vi "Dashboard Main.vi"() -> ()   [LabVIEW 2016]
uses:
  <vilib>/Utility/miscctls.llb/LVRowAndColumnTypeDef.ctl
  <vilib>/event_ctls.llb/eventvkey.ctl
  <vilib>/Rock Robotics/Network Tables/NT Read Numeric Array.vi
  <vilib>/Rock Robotics/Network Tables/NT Read Boolean.vi
  <vilib>/Rock Robotics/Network Tables/NT Write Boolean.vi
  <vilib>/Rock Robotics/Network Tables/NT Read Boolean Array.vi
  <vilib>/Utility/file.llb/Read Delimited Spreadsheet (string).vi
  <vilib>/Utility/file.llb/Read Delimited Spreadsheet (DBL).vi
  <vilib>/Rock Robotics/Network Tables/NT Write String Array.vi
  <vilib>/Utility/file.llb/Write Delimited Spreadsheet (string).vi
  <vilib>/Rock Robotics/Network Tables/NT Write Numeric Array.vi
  <vilib>/Utility/file.llb/Write Delimited Spreadsheet (DBL).vi
  <vilib>/Rock Robotics/WPI/Dashboard/WPI_DashboardLogging Global.vi
panel:
  in  "Camera Settings Right":T1={"Frame Rate"=15, "Compression"=30, "Size"=1, "DB Camera Config"=FALSE} {"Frame Rate" scale=1.0..30.0; "Compression" scale=100.0..-1.0; "Size" items=["640x480", "320x240", "160x120"]}
  in  "Camera Name Right":string(combo)="No Camera Selection"
  out "Camera Info":cluster{"Mbps LED":bool, "Mbps":dbl, "fps":dbl} {"fps" format="%#.1g"; "Mbps" format="%#.1g"}
  in  "Camera Settings":T1={"Frame Rate"=15, "Compression"=30, "Size"=1, "DB Camera Config"=FALSE} {"Frame Rate" scale=1.0..30.0; "Compression" scale=100.0..-1.0; "Size" items=["640x480", "320x240", "160x120"]}
  in  "TCP":refnum<k5>
  in  "Rec Mode":enum32{"Stop", "Record", "Playback"}(radio)
  out "Robot IP":string="0.0.0.0"
  out "Image Message":string="Timeout in Camera Communications"
  in  "Dashboard Tab":T2(tab)=enum."Config"
  in  "Disable Drop Ropes":bool
  out "Shoot RPM":dbl format="%#_10f"
  in  "Config File Path":path=path "C:/Users/Admin/Desktop/ConfigCSV.csv"
  in  "Slow Drive":dbl=50.0
  in  "Fast Drive":dbl=100.0
  out "Shoot PWM":dbl
  in  "Thump Interval":dbl=0.4
  out "Pixy Height":dbl
  out "Pixy Width":dbl
  out "Pixy X":dbl
  in  "Lock Servo B":dbl=170.0
  in  "Lock Servo A":dbl
  out "Move":dbl=85.0
  out "Zero":dbl=77.0
  in  "Gear Servo Values":u16(ring) items=["A Values | Comp", "B Values | Practice"]
  in  "Gear Servo Move B":dbl=85.0
  in  "Gear Servo Move A":dbl=85.0
  in  "Gear Servo Zero B":dbl=79.5
  in  "Gear Servo Zero A":dbl=77.0
  out "Notify 2":string="NT Disconnected"
  out "Verify 2":string="No Comm"
  in  "Time Remain":bool=TRUE
  out "Auto Ran":string="Not Available"
  out "Code Version":string="Not Available"
  out "NT Connection":bool
  out "MotorChart R":cluster{"Numeric":dbl, "Numeric":dbl}(graph)
  out "MotorChart L":cluster{"Numeric":dbl, "Numeric":dbl}(graph)
  out "MotorSliders R":cluster{"MotorSlide1":dbl, "MotorSlide2":dbl} {"MotorSlide2" scale=-1.0..1.0 scale format="%#_2e"; "MotorSlide1" scale=-1.0..1.0 scale format="%#_2e"}
  out "MotorSliders L":cluster{"MotorSlide1":dbl, "MotorSlide2":dbl} {"MotorSlide2" scale=-1.0..1.0 scale format="%#_2e"; "MotorSlide1" scale=-1.0..1.0 scale format="%#_2e"}
  out "JS1 Z":dbl(slide) scale=-1.0..1.0 scale format="%#_2e"
  out "JS1 Graph":cluster{"X":dbl, "Y":dbl}[](graph)
  out "JS1 Buttons":T3
  out "JS2 Z":dbl(slide) scale=-1.0..1.0 scale format="%#_2e"
  out "JS2 Graph":cluster{"X":dbl, "Y":dbl}[](graph)
  out "JS2 Buttons":T3
  out "Mode":T4(ring)=enum."Disconnected"
  in  "Auto Array File Path":path=path "C:/Users/Admin/Desktop/AutoCSV.csv"
  out "Camera Image Right":T5(plugin-control)
  out "Climb Inverted":bool
  in  "Auto Gear Timeout":dbl=-1.0
  out "Shoot Toggle":bool
  in  "Auto Turn Speed":dbl=0.4
  out "Gear Box Stat":bool
  in  "Auto Drive Speed":dbl=0.5
  in  "RPM 4":dbl=0.85
  in  "RPM 3":dbl=0.95
  in  "RPM 2":dbl=0.9
  in  "Serializer Speed":dbl=0.8
  out "Gear Plate":bool
  in  "Pixy Center":dbl=-2.3
  in  "RPM 1":dbl=1.0 min=0.0 max=1.0
  in  "Climb Speed":dbl=1.0
  in  "Slow Turn":dbl=50.0
  in  "Fast Turn":dbl=100.0
  in  "Auto Select":string(combo)="Default"
  out "Pixy Object Stat":bool
  out "Time Remaining":dbl=135.0 format="%#.0f"
  out "PDP Comm":string="Code Ver : Not Available"
  out "PDP Comm":bool=TRUE
  out "Notifyer":bool
  out "Notifyer Box":string="ERROR - DS is not Running"
  out "Auto Ready":bool
  out "Verify":string="Auto Ran : Not Available"
  in  "Position":string(combo)="Default"
  out "Gear Status":bool
  out "Channel 8":bool
  out "Channel 7":bool
  out "Channel 6":bool
  out "Channel 5":bool
  out "Channel 10":bool
  out "Channel 9":bool
  out "Channel 4":bool
  out "Channel 11":bool
  out "Channel 3":bool
  out "Channel 1":bool
  out "Channel 0":bool
  out "Channel 2":bool
  out "Channel 11":dbl
  out "Channel 10":dbl
  out "Channel 9":dbl
  out "Channel 8":dbl
  out "Channel 7":dbl
  out "Channel 6":dbl
  out "Channel 5":dbl
  out "Channel 4":dbl
  out "Channel 3":dbl
  out "Channel 2":dbl
  out "Channel 1":dbl
  out "Channel 15":bool
  out "Channel 14":bool
  out "Channel 13":bool
  out "Channel 12":bool
  out "Channel 15":dbl
  out "Channel 14":dbl
  out "Channel 13":dbl
  out "Channel 12":dbl
  out "Channel 0":dbl
  in  "Reset Sticky":bool
  in  "Reset Latched":bool
  out "Config Saved":bool
  in  "Update Config":bool
  in  "ARM Write":bool
  in  "Read Config":bool
  in  "Config Cluster":T6={"a"=0.0, "b"=0.0, "c"=0.0, "d"=0.0, "h"=0.0, "proportional gain (Kc)"=0.019, "integral time (Ti, min)"=0.0, "derivative time (Td, min)"=0.0, "Fast Speed"=-0.3, "setpoint"=1400.0, "Approach Speed"=-0.12, "proportional gain (Kc) 2"=0.052, "integral time (Ti, min) 2"=0.0, "derivative time (Td, min) 2"=0.002, "Cutoff Delay"=0.5, "Sense Delay"=0.0, "Wait Till Shoot"=0.0, "proportional gain (Kc) 3"=0.0, "integral time (Ti, min) 3"=0.0, "derivative time (Td, min) 3"=0.0, "Aim Offset"=0.0, "PWM Offset"=0.0} {"derivative time (Td, min) 3" format="%.3f"; "integral time (Ti, min) 3" format="%.3f"; "proportional gain (Kc) 3" format="%.3f"; "Cutoff Delay" min=0.0; "derivative time (Td, min)" format="%.3f"; "integral time (Ti, min)" format="%.3f"; "proportional gain (Kc)" format="%.3f"; "derivative time (Td, min) 2" format="%.3f"; "integral time (Ti, min) 2" format="%.3f"; "proportional gain (Kc) 2" format="%.3f"}
  in  "Test Slider":dbl(slide) scale=0.0..100.0 scale format="%#_3g"
  in  "On/Off":bool caption="Solenoid"
  in  "Test Name":u16(ring) items=["Select the test to run..."]
  in  "Test Tree":string(tree)
  in  "Motor":cluster{"Value":dbl, "Enable":bool} {"Value" scale=-1.0..1.0 scale format="%#_3g"}
  out "Progress":T7 {"Test Progress" scale=0.0..100.0}
  in  "Rev/Fwd":cluster{"Forward":bool, "Reverse":bool}
  in  "Test Ring":u16(ring) items=["Monochrome", "Color"]
  out "Cmd Status":string
  in  "Execute Command":bool
  in  "Command Params":string[][](table)
  in  "Command Selection":i32(listbox)
  out "Saved to Sheet":bool
  in  "ARM Overwrite":bool
  in  "Read Sheet":bool
  in  "Update Sheet":bool
  in  "Auto Array":string[][](array[string])
  in  "CheckList":i32(listbox)
  out "Tree":string(tree)
  out "Camera Image":T5(plugin-control)
  out "Background":bool
  in  "Camera Name":string(combo)="No Camera Selection"
  # "HW"
  # "HW"
  # "Joysticks"
  # "Drive Motors"
  # "Front"
  # "Right"
  # "Left"
  # "Back"
  # "Manual PWM"
  # "Drivetrain"
  # "Shooter"
  # "Climbing"
  # "Serializer"
  # "Unused"
  # "Feeder"
  # "Intake"
  # "Shooting Coefficents"
  # "Gear Aiming PID Gains"
  # "Other Gear Aiming Stuff"
  # "Shooting Aiming PID Gains"
  # "Other Shooting Stuff"
  # "More Shooting Stuff"
  # "Shoot Wheel PID Gains"
  # "Format: [Command] [Time in Tenths]"
  # "Label         Move 1       Rot 1         Act 1        Move 2       Rot 2        Move 3       Act 2"
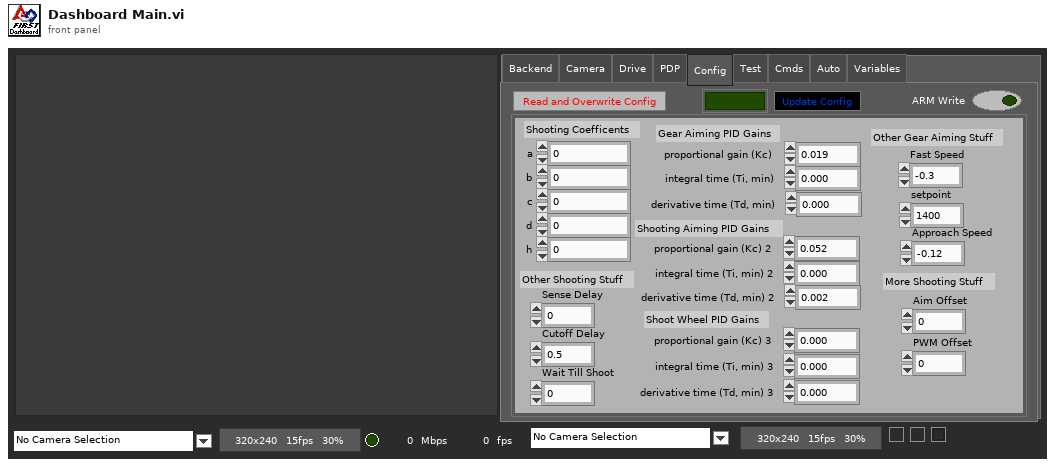
[diagram p1: front panel]
types:
  T1 = cluster{"Frame Rate":i32, "Compression":i32, "Size":u16, "DB Camera Config":bool}
  T2 = enum32{"Backend", "Camera", "Drive", "PDP", "Config", "Test", "Cmds", "Auto", "Variables"}
  T3 = cluster{bool, bool, bool, bool, bool, bool, bool, bool, bool, bool, bool, bool}
  T4 = enum8{"Tele-Op Disabled", "Tele-Op Enabled", "Auto Disabled", "Auto Enabled", "Test Disabled", "Test Enabled", "Disconnected", "No Code", "E-Stop"}
  T5 = typedef "IMAQ Image.ctl" = refnum<image>
  T6 = cluster{"a":dbl, "b":dbl, "c":dbl, "d":dbl, "h":dbl, "proportional gain (Kc)":dbl, "integral time (Ti, min)":dbl, "derivative time (Td, min)":dbl, "Fast Speed":dbl, "setpoint":dbl, "Approach Speed":dbl, "proportional gain (Kc) 2":dbl, "integral time (Ti, min) 2":dbl, "derivative time (Td, min) 2":dbl, "Cutoff Delay":dbl, "Sense Delay":dbl, "Wait Till Shoot":dbl, "proportional gain (Kc) 3":dbl, "integral time (Ti, min) 3":dbl, "derivative time (Td, min) 3":dbl, "Aim Offset":dbl, "PWM Offset":dbl}
  T7 = cluster{"Test Progress":u8, "Test Progress Text":string}
  T8 = typedef "Image Type" = u32
  T9 = cluster{"IDs":cluster{"RPC field ID":u16, "Unique ID":u16}, "String":string}
  T10 = enum32{"Drive", "Basic", "Custom", "Test", "Checklist", "Variables"}
  T11 = cluster{"all rows[0]":dbl, "all rows[1]":dbl, "all rows[2]":dbl, "all rows[3]":dbl, "all rows[4]":dbl, "all rows[5]":dbl, "all rows[6]":dbl, "all rows[7]":dbl, "all rows[8]":dbl, "all rows[9]":dbl, "all rows[10]":dbl, "all rows[11]":dbl, "all rows[12]":dbl, "all rows[13]":dbl, "all rows[14]":dbl, "all rows[15]":dbl, "all rows[16]":dbl, "all rows[17]":dbl, "all rows[18]":dbl, "all rows[19]":dbl, "all rows[20]":dbl, "all rows[21]":dbl}
  T12 = cluster{"Error Strings":string, "Disable Counts":cluster{u16, u16}, "Rail Faults":cluster{u16, u16, u16}, "Robot IP":string, "DB Mode":u8, "Event Info":cluster{"Name":string, "Type":u8, "Number":u16, "Replay":u8}}
  T13 = cluster{"Storage":cluster{"Disk Free":u64, "RAM Block":u32, "RAM free":u32}, "CPU Utilization":cluster{"CPU % ISR":sgl, "CPU % Time Crit":sgl, "CPU % Timed Str":sgl, "CPU % High":sgl, "CPU % Above":sgl, "CPU % Normal":sgl, "CPU % Low":sgl}, "CAN":cluster{"% Bus Utilization":sgl, "Bus Off Cnt":u32, "TX_FIFO Full Cnt":u32, "Receive Error Cnt":u8, "Transmit Error Cnt":u8}, "HID":cluster{"HID Outputs":u32, "Rumble Low":u16, "Rumble High":u16}[]}
  T14 = cluster{"Status bits":cluster{"Test Mode":bool, "Autonomous":bool, "Enabled":bool, "Code Start":bool, "Brownout":bool, "Reserved 2":bool, "Reserved 3":bool, "E-Stop":bool}, "Code Trace":cluster{"Disabled":bool, "TeleOp":bool, "Auto":bool, "Test":bool}, "Controller Type":enum16{"unknown", "cRIO", "roboRio"}, "Code?":enum16{"unknown", "noCode", "code"}, "Battery V":dbl}
  T15 = cluster{"Control Bits":cluster{"TestMode":bool, "Autonomous":bool, "Enabled":bool, "FMS Present":bool, bool, bool, bool, "E-Stop":bool}, "Team Station ":u8, "Countdown":sgl, "Joystick Values":cluster{"Axes":dbl[], "Buttons":bool[], "POVs":i16[]}[]}
  T16 = cluster{"Axes":dbl[], "Buttons":bool[], "POVs":i16[]}[]
  T17 = cluster{"Axes":dbl[], "Buttons":bool[], "POVs":i16[]}
  T18 = cluster{"Buttons[0]":bool, "Buttons[1]":bool, "Buttons[2]":bool, "Buttons[3]":bool, "Buttons[4]":bool, "Buttons[5]":bool, "Buttons[6]":bool, "Buttons[7]":bool, "Buttons[8]":bool, "Buttons[9]":bool, "Buttons[10]":bool, "Buttons[11]":bool}
  T19 = cluster{"Camera Image":refnum<vi>, "Dashboard Tab":refnum<vi>, "Background":refnum<vi>, "Rec Mode":refnum<vi>, "Test Slider":refnum<vi>, "On/Off ":refnum<vi>, "Test Ring":refnum<vi>, "Rev/Fwd":refnum<vi>, "Test Name":refnum<vi>, "Motor":refnum<vi>, "Progress":refnum<vi>, "CheckList":refnum<vi>, "Tree":refnum<vi>, "Test Tree":refnum<vi>, "Command Params":refnum<vi>, "Command Selection":refnum<vi>, "Execute Command":refnum<vi>, "Cmd Status":refnum<vi>, "Camera Settings":refnum<vi>, "Camera Name":refnum<vi>, "Camera Info":refnum<vi>, "Camera Settings Right":refnum<vi>, "Camera Name Right":refnum<vi>, "Camera Image Right":refnum<vi>}
  T20 = cluster{"Operation":enum16{"Update", "Clear"}, "Color Box":u32}[]
  T21 = typedef "eventvkey.ctl" = enum16{"ASCII", "Enter", "Return", "Shift", "Ctrl", "Alt", "Cmd", "Opt", "Caps", "NumLock", "Clear", "Break", "Up", "Down", "Left", "Right", "Insert", "Delete", "Home", "End", "PageUp", "PageDown", "Escape", "Help", "Pause", "ScrollLock", "F1", "F2", "F3", "F4", "F5", "F6", "F7", "F8", "F9", "F10", "F11", "F12", "F13", "F14", "F15", "F16", "F17", "F18", "F19", "F20", "F21", "F22", "F23", "F24", "Play", "VolumeUp", "VolumeDown", "Mute", "Two Byte Char"}
  T22 = cluster{"Image Size":bool, "Image Type":bool, "Pixel Value":bool, "ROI Information":bool, "Zoom Factor":bool}
  T23 = cluster{"Operation":enum16{"Update", "Clear"}, "Color Box":u32}
  T24 = typedef "LVRowAndColumnTypeDef.ctl" = cluster{"Row":i32, "Column":i32}
  T25 = cluster{"Shift":bool, "Ctrl":bool, "Alt":bool, "Cmd":bool, "Opt":bool}
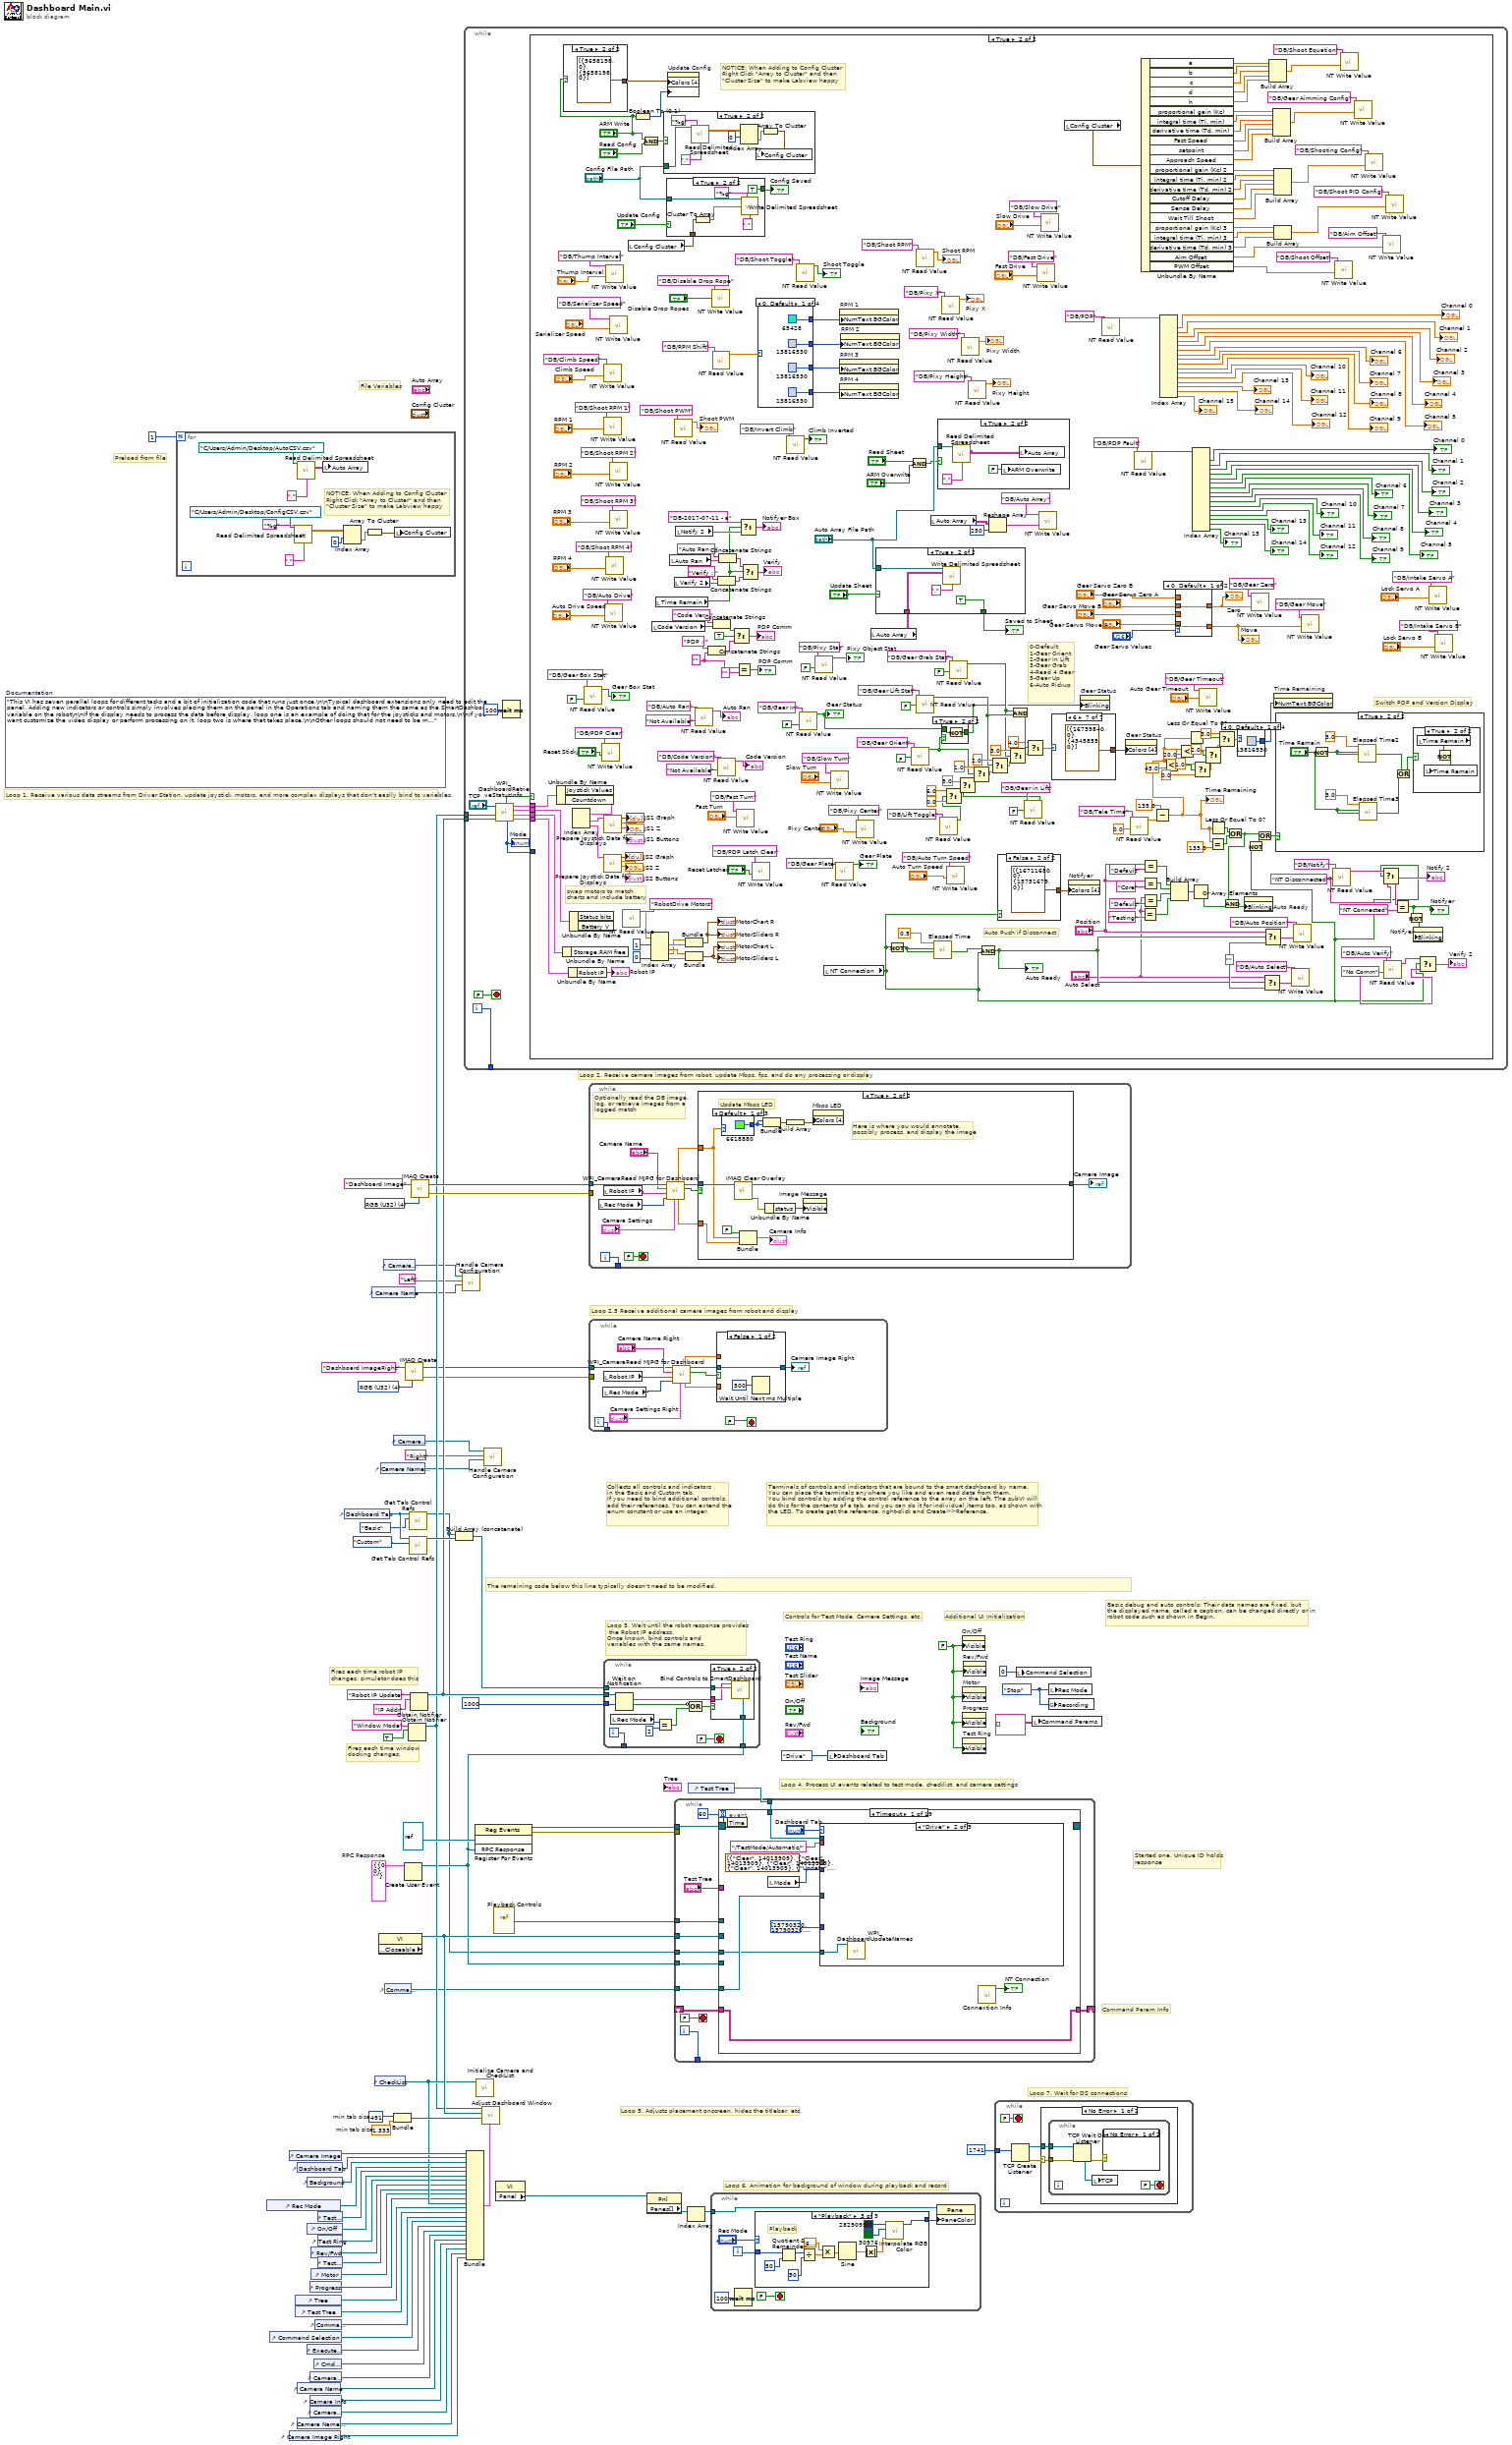
[diagram p0: block diagram]
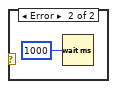
[diagram p3: hidden frame]
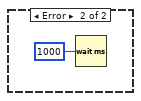
[diagram p4: hidden frame]
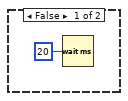
[diagram p5: hidden frame]
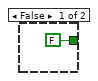
[diagram p6: hidden frame]
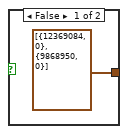
[diagram p7: hidden frame]
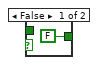
[diagram p9: hidden frame]
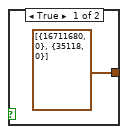
[diagram p10: hidden frame]
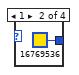
[diagram p12: hidden frame]
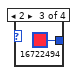
[diagram p13: hidden frame]
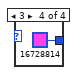
[diagram p14: hidden frame]
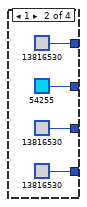
[diagram p15: hidden frame]
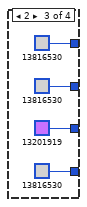
[diagram p16: hidden frame]
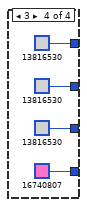
[diagram p17: hidden frame]
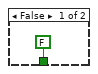
[diagram p19: hidden frame]
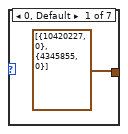
[diagram p20: hidden frame]
diagram:
  w11 = T8 4 items=["Grayscale (U8)", "Grayscale (I16)", "Grayscale (SGL)", "Complex (CSG)", "RGB (U32)", "HSL (U32)", "RGB (U64)"] ("Image Type")
  w25 = T9 {"IDs"={"RPC field ID"=0, "Unique ID"=0}, "String"=""}  # RPC Response
  w50 = 491  # min tab size
  w49 = 1.333  # min tab size
  w57 = enum32{"Stop", "Record", "Playback"}."Stop" ("Rec Mode")
  w32 = FALSE ("Visible")
  (unwired) "This VI has seven parallel loops for different tasks and a bit of initialization code that runs just once.\n\nTypical dashboard extensions only need to edit the panel. Adding new indicators or controls simply involves placing them on the panel in the Operations tab and naming them the same as the SmartDashboard variable on the robot\n\nIf the display needs to process the data before display, loop one is an example of doing that for the joysticks and motors.\n\nIf you want customize the video display or perform processing on it, loop two is where that takes place.\n\nOther loops should not need to be modified. They are pretty standard, and document the task they perform."  # Documentation
  w74 = T8 4 items=["Grayscale (U8)", "Grayscale (I16)", "Grayscale (SGL)", "Complex (CSG)", "RGB (U32)", "HSL (U32)", "RGB (U64)"] ("Image Type")
  # "File Variables"
  # "Preload from file"
  # "Loop 2.5 Receive additional camera images from robot and display"
  # "Command Param Info"
  # "Started one, Unique ID holds\nresponse"
  # "Loop 7. Wait for DS connections"
  # "Basic debug and auto controls: Their data names are fixed, but\nthe displayed name, called a caption, can be changed directly or in\nrobot code such as shown in Begin."
  # "Controls for Test Mode, Camera Settings, etc."
  # "Additional UI Initialization"
  # "Loop 6. Animation for background of window during playback and record"
  # "Fires each time robot IP\nchanges, simulator does this"
  # "Fires each time window\ndocking changes."
  # "Collects all controls and indicators\nin the Basic and Custom tab.\nIf you need to bind additional controls,\nadd their references. You can extend the\nenum constant or use an integer."
  # "The remaining code below this line typically doesn't need to be modified."
  # "Loop 4. Process UI events related to test mode, checklist, and camera settings"
  # "Terminals of controls and indicators that are bound to the smart dashboard by name.\nYou can place the terminals anywhere you like and even read data from them.\nYou bind controls by adding the control reference to the array on the left. The subVI will\ndo this for the contents of a tab, and you can do it for individual items too, as shown with\nthe LED. To create get the reference, right-click and Create>>Reference."
  # "Loop 3. Wait until the robot response provides\n the Robot IP address.\nOnce known, bind controls and\nvariables with the same names."
  # "Loop 5. Adjusts placement onscreen, hides the titlebar, etc."
  # "Loop 1. Receive various data streams from Driver Station, update joystick, motors, and more complex displays that don't easily bind to variables."
  # "Loop 2. Receive camera images from robot, update Mbps, fps, and do any processing or display"
  n1 = for {
    N: 1 -> [_]
    # "NOTICE: When Adding to Config Cluster\nRight Click \"Array to Cluster\" and then \n\"Cluster Size\" to make Labview happy"
    n2 = call-poly <vilib>:"Read Delimited Spreadsheet.vi"("file path (dialog if empty)"=path "C:/Users/Admin/Desktop/ConfigCSV.csv", "format (%.3f)"="%g", "delimiter (\\t)"="," ("delimiter (\\t)")) -> ("all rows"=w79:dbl[][])  [unwired: 7 in, 5 out]
    n3 = call-poly <vilib>:"Read Delimited Spreadsheet.vi"("file path (dialog if empty)"=path "C:/Users/Admin/Desktop/AutoCSV.csv", "delimiter (\\t)"="," ("delimiter (\\t)")) -> ("all rows"=w82:string[][])  [unwired: 8 in, 5 out]
    n4 = local write "Auto Array"(w82) -> ()
    n5 = Index Array(array=w79, index (row)=0 ("disabled index (col)")) -> (element=w78:dbl[])  [unwired: 1 in]
    n6 = Array To Cluster(array=w78) -> (cluster=w75:T11)
    n7 = local write "Config Cluster"(w75) -> ()
  }
  n8 = control-ref of="Rec Mode"() -> (w38:refnum<vi>)
  n9 = control-ref of="Command Selection"() -> (w24:refnum<vi>)
  n10 = control-ref of="Camera Image Right"() -> (w2:refnum<vi>)
  n11 = control-ref of="Camera Image"() -> (w52:refnum<vi>)
  n12 = control-ref of="Tree"() -> (w42:refnum<vi>)
  n13 = control-ref of="Test Tree"() -> (w41:refnum<vi>)
  n14 = control-ref of="Dashboard Tab"() -> (w51:refnum<vi>)
  n15 = control-ref of="Camera Name"() -> (w15:refnum<vi>)
  n16 = control-ref of="Camera Name Right"() -> (w3:refnum<vi>)
  n17 = control-ref of="Execute Command"() -> (w26:refnum<vi>)
  n18 = control-ref of="Background"() -> (w47:refnum<vi>)
  n19 = control-ref of="On/Off"() -> (w36:refnum<vi>)
  n20 = control-ref of="Progress"() -> (w33:refnum<vi>)
  n21 = control-ref of="Camera Settings"() -> (w16:refnum<vi>)
  n22 = control-ref of="Camera Info"() -> (w14:refnum<vi>)
  n23 = control-ref of="Camera Settings Right"() -> (w4:refnum<vi>)
  n24 = control-ref of="Rev/Fwd"() -> (w34:refnum<vi>)
  n25 = control-ref of="Motor"() -> (w39:refnum<vi>)
  n26 = control-ref of="Cmd Status"() -> (w20:refnum<vi>)
  n27 = control-ref of="Command Params"() -> (w27:refnum<vi>)
  n28 = control-ref of="Test Slider"() -> (w37:refnum<vi>)
  n29 = control-ref of="Test Ring"() -> (w35:refnum<vi>)
  n30 = control-ref of="Test Name"() -> (w40:refnum<vi>)
  n31 = control-ref of="Dashboard Tab"() -> (w55:refnum<vi>)
  n32 = control-ref of="Camera Name"() -> (w17:refnum<vi>)
  n33 = control-ref of="CheckList"() -> (w43:refnum<vi>)
  n34 = property class="VI" props=["Front Panel.Closeable"]() -> (reference out=w56:refnum<vi>)  [unwired: 2 in, 2 out]
  n35 = control-ref of="Camera Name Right"() -> (w7:refnum<vi>)
  n36 = control-ref of="Camera Settings"() -> (w18:refnum<vi>)
  n37 = control-ref of="Command Params"() -> (w19:refnum<vi>)
  n38 = control-ref of="Camera Settings Right"() -> (w8:refnum<vi>)
  n39 = Bundle("min tab size"=w50, "min tab size"=w49) -> (w48:cluster{"min tab size":i32, "min tab size":dbl})  [unwired: 1 in]
  n40 = Create User Event(user event datatype=w25) -> (user event=w21:refnum<user-event>)  [unwired: 1 in, 1 out]
  n41 = call "IMAQ Create"("Image Name"="Dashboard ImageRight", "Image Type"=w11) -> ("New Image"=w10:T5, "error out"=w9:errorcluster)  [unwired: 2 in, 1 out]
  n42 = Obtain Notifier(name (unnamed)="Window Mode", notification data type=TRUE) -> (notifier out=w30:refnum<notifier>)  [unwired: 2 in, 2 out]
  n43 = call <vilib>:"Get Tab Control Refs.vi"("Page Index"=T10."Basic" ("Dashboard Tab"), "TabControl in"=w55) -> ("ControlsOnPage"=w13:refnum<vi>[])  [unwired: 9 in]
  n44 = call <vilib>:"Get Tab Control Refs.vi"("Page Index"=T10."Custom" ("Dashboard Tab"), "TabControl in"=w55) -> ("ControlsOnPage"=w54:refnum<vi>[])  [unwired: 9 in]
  n45 = Obtain Notifier(name (unnamed)="Robot IP Update", notification data type="IP Addr" ("name (unnamed)")) -> (notifier out=w31:refnum<notifier>)  [unwired: 2 in, 2 out]
  n46 = call "IMAQ Create"("Image Name"="Dashboard Image", "Image Type"=w74) -> ("New Image"=w72:T5, "error out"=w71:errorcluster)  [unwired: 2 in, 1 out]
  n47 = Build Array (concatenate)(w13, w54) -> (w53:refnum<vi>[])
  n48 = call "Handle Camera Configuration.vi"("CameraNameRef"=w17, "Camera File Name"="Left", "ClusterRef"=w18) -> ()  [unwired: 9 in]
  n49 = while {
    tunnel: [w95] -> _
    tunnel: w31 -> [w89]
    tunnel: w30 -> [w86]
    i -> [w95]
    stop <- FALSE stop-if-true
    n50 = call <vilib>:"WPI_DashboardRetrieveStatusInfo.vi"("Binding Refnum"=w89, "Window Mode Notifier"=w86, "TCP Cnx"="TCP") -> ("Power and Errors"=w90:T12, "Robot Metrics"=w93:T13, "Status Info"=w94:T14, "Control Info"=w91:T15, "Robot Mode"=w88:T4, "Process?"=w92:bool)  [unwired: 3 in]
    "Mode" <- w88
    n51 = Wait (ms)(milliseconds to wait=u32 100) -> ()  [unwired: 1 out]
    n52 = case shown="True" w92 {
      tunnel: w94 -> [_ w406]
      tunnel: w93 -> [_ w405]
      tunnel: w91 -> [_ w404]
      tunnel: w90 -> [_ w403]
      tunnel: w88 -> [_ _]
      frame False {
        n53 = Wait (ms)(milliseconds to wait=u32 20) -> ()  [unwired: 1 out]
      }
      frame True {
        w303 = ""
        w343 = "NT Disconnected" ("Default Value")
        w370 = "No Comm" ("Default Value")
        w375 = ""
        # "0-Default\n1-Gear Orient\n2-Gear In Lift\n3-Gear Grab\n4-Read 4 Gear\n5-Gear Up\n6-Auto Pickup"
        # "NOTICE: When Adding to Config Cluster\nRight Click \"Array to Cluster\" and then \n\"Cluster Size\" to make Labview happy"
        # "Switch PDP and Version Display"
        # "Auto Push if Disconnect"
        # "swap motors to match\ncharts and include battery"
        n54 = Unbundle By Name(w404) -> ("Joystick Values"=w394:T16)  [unwired: 1 out]
        n55 = Unbundle By Name(w405) -> ()  [unwired: 1 out]
        n56 = case shown="True" "ARM Write" {
          tunnel: [cluster{u32, u32}[] [{12369084, 0}, {9868950, 0}] ("Colors [4]") cluster{u32, u32}[] [{5658198, 0}, {5658198, 0}] ("Colors [4]")] -> w145
          frame False {
          }
          frame True {
          }
        }
        n57 = Unbundle By Name(w403) -> ("Robot IP"=→"Robot IP":string)
        n58 = Unbundle By Name(w406) -> ()  [unwired: 2 out]
        n59 = Index Array(array=w394) -> (element #1=w393:T17, element #2=w389:T17)  [unwired: 2 in]
        n60 = call-poly <vilib>:"NT Read Value.vi"("Default Value"=FALSE, "Name"="DB/Gear Box Stat") -> ("Boolean"=→"Gear Box Stat":bool)  [unwired: 8 in, 1 out]
        n61 = call-poly <vilib>:"NT Write Value.vi"("Boolean"="Reset Sticky", "Name"="DB/PDP Clear") -> ()  [unwired: 9 in, 1 out]
        n62 = call-poly <vilib>:"NT Write Value.vi"("Numeric"="Climb Speed", "Name"="DB/Climb Speed") -> ()  [unwired: 9 in, 1 out]
        n63 = call "Prepare Joystick Data for Displays.vi"("Joystick Values"=w389) -> ("Buttons"=→"JS2 Buttons":T18, "Z Axis"=→"JS2 Z":dbl, "Cartesian Data"=→"JS2 Graph":cluster{"X axis":dbl, "X axis":dbl}[])  [unwired: 8 in]
        n64 = call-poly <vilib>:"NT Write Value.vi"("Numeric"="RPM 1", "Name"="DB/Shoot RPM 1") -> ()  [unwired: 9 in, 1 out]
        n65 = call "Prepare Joystick Data for Displays.vi"("Joystick Values"=w393) -> ("Buttons"=→"JS1 Buttons":T18, "Z Axis"=→"JS1 Z":dbl, "Cartesian Data"=→"JS1 Graph":cluster{"X axis":dbl, "X axis":dbl}[])  [unwired: 8 in]
        n66 = call-poly <vilib>:"NT Write Value.vi"("Numeric"="Auto Drive Speed", "Name"="DB/Auto Drive") -> ()  [unwired: 9 in, 1 out]
        n67 = call-poly <vilib>:"NT Write Value.vi"("Numeric"="Thump Interval", "Name"="DB/Thump Interval") -> ()  [unwired: 9 in, 1 out]
        n68 = call-poly <vilib>:"NT Write Value.vi"("Numeric"="RPM 4", "Name"="DB/Shoot RPM 4") -> ()  [unwired: 9 in, 1 out]
        n69 = call-poly <vilib>:"NT Write Value.vi"("Numeric"="Serializer Speed", "Name"="DB/Serializer Speed") -> ()  [unwired: 9 in, 1 out]
        n70 = call-poly <vilib>:"NT Write Value.vi"("Numeric"="RPM 2", "Name"="DB/Shoot RPM 2") -> ()  [unwired: 9 in, 1 out]
        n71 = call-poly <vilib>:"NT Write Value.vi"("Numeric"="RPM 3", "Name"="DB/Shoot RPM 3") -> ()  [unwired: 9 in, 1 out]
        n72 = call-poly <vilib>:"NT Read Value.vi"("Name"="RobotDrive Motors") -> ("Numeric Array"=w384:dbl[])  [unwired: 9 in, 1 out]
        n73 = local read "Config Cluster"() -> (w141:T6)
        n74 = Boolean To (0,1)(Boolean="ARM Write") -> (0, 1=w146:i16)
        n75 = And(x="ARM Write", y="Read Config") -> (x .and. y?=w148:bool)
        n76 = Index Array(array=w384, index #1=1, index #4=0) -> (element #1=w398:dbl, element #2=w399:dbl, element #3=w397:dbl, element #4=w402:dbl)  [unwired: 2 in]
        n77 = local read "Code Version"() -> (w305:string)
        n78 = local read "Time Remain"() -> (w298:bool)
        n79 = case shown="True" w148 {
          tunnel: "Config File Path" -> [_ w419]
          frame False {
          }
          frame True {
            n80 = call-poly <vilib>:"Read Delimited Spreadsheet.vi"("file path (dialog if empty)"=w419, "format (%.3f)"="%g", "delimiter (\\t)"="," ("delimiter (\\t)")) -> ("all rows"=w421:dbl[][])  [unwired: 7 in, 5 out]
            n81 = Index Array(array=w421, index (row)=0 ("disabled index (col)")) -> (element=w422:dbl[])  [unwired: 1 in]
            n82 = Array To Cluster(array=w422) -> (cluster=w416:T11)
            n83 = local write "Config Cluster"(w416) -> ()
          }
        }
        n84 = case shown="True" "Update Config" {
          tunnel: "Config File Path" -> [_ w413]
          tunnel: w141 -> [_ w411]
          tunnel: [FALSE TRUE] -> w140
          frame False {
          }
          frame True {
            n85 = Cluster To Array(cluster=w411) -> (array=w410:dbl[])
            n86 = call-poly <vilib>:"Write Delimited Spreadsheet.vi"("file path (dialog if empty)"=w413, "format (%.3f)"="%g", "1D data"=w410, "delimiter (\\t)"="," ("delimiter (\\t)")) -> ()  [unwired: 10 in, 2 out]
          }
        }
        "Config Saved" <- w140
        n87 = property on="Update Config" class="Bool"("Colors [4]"=w145, "DisabledEnum"=w146) -> ()  [unwired: 2 in, 2 out]
        n88 = local read "Auto Ran"() -> (w309:string)
        n89 = local read "Verify 2"() -> (w307:string)
        n90 = call-poly <vilib>:"NT Read Value.vi"("Name"="DB/Shoot PWM") -> ("Numeric"=→"Shoot PWM":dbl)  [unwired: 9 in, 1 out]
        n91 = local read "Notify 2"() -> (w299:string)
        n92 = Bundle("Numeric"=w397, "Numeric"=w398) -> (→"MotorChart R" →"MotorSliders R":cluster{"Numeric":dbl, "Numeric":dbl})  [unwired: 1 in]
        n93 = Bundle("Numeric"=w399, "Numeric"=w402) -> (→"MotorChart L" →"MotorSliders L":cluster{"Numeric":dbl, "Numeric":dbl})  [unwired: 1 in]
        n94 = call-poly <vilib>:"NT Read Value.vi"("Default Value"="Not Available", "Name"="DB/Auto Ran") -> ("String"=→"Auto Ran":string)  [unwired: 8 in, 1 out]
        n95 = Concatenate Strings("PDP : " ("string"), w303) -> (w302:string)
        n96 = call-poly <vilib>:"NT Write Value.vi"("Boolean"="Disable Drop Ropes", "Name"="DB/Disable Drop Rope") -> ()  [unwired: 9 in, 1 out]
        n97 = call-poly <vilib>:"NT Read Value.vi"("Name"="DB/RPM Shift") -> ("Numeric"=w275:dbl)  [unwired: 9 in, 1 out]
        n98 = Concatenate Strings("Code Ver : " ("string"), w305) -> (w304:string)
        n99 = call-poly <vilib>:"NT Read Value.vi"("Default Value"="Not Available", "Name"="DB/Code Version") -> ("String"=→"Code Version":string)  [unwired: 8 in, 1 out]
        n100 = Concatenate Strings("Verify : " ("string"), w307) -> (w306:string)
        n101 = Concatenate Strings("Auto Ran : " ("string"), w309) -> (w308:string)
        n102 = Select(t=w304, s=TRUE, f=w302) -> (s? t:f=→"PDP Comm":string)
        n103 = Equal?(x=w303, y="") -> (x = y?=→"PDP Comm":bool)
        n104 = call-poly <vilib>:"NT Write Value.vi"("Numeric"="Fast Turn", "Name"="DB/Fast Turn") -> ()  [unwired: 9 in, 1 out]
        n105 = Select(t="DB-2017-07-11 - a" ("string"), s=w298, f=w299) -> (s? t:f=→"Notifyer Box":string)
        n106 = Select(t=w308, s=w298, f=w306) -> (s? t:f=→"Verify":string)
        n107 = call-poly <vilib>:"NT Write Value.vi"("Boolean"="Reset Latched", "Name"="DB/PDP Latch Clear") -> ()  [unwired: 9 in, 1 out]
        n108 = case shown="0, Default" w275 {
          tunnel: [u32 65428 u32 13816530 u32 13816530 u32 13816530] -> w274
          tunnel: [u32 13816530 u32 54255 u32 13816530 u32 13816530] -> w273
          tunnel: [u32 13816530 u32 13816530 u32 13201919 u32 13816530] -> w272
          tunnel: [u32 13816530 u32 13816530 u32 13816530 u32 16740807] -> w271
          frame 0, Default {
          }
          frame 1 {
          }
          frame 2 {
          }
          frame 3 {
          }
        }
        n109 = call-poly <vilib>:"NT Read Value.vi"("Name"="DB/Invert Climb") -> ("Boolean"=→"Climb Inverted":bool)  [unwired: 9 in, 1 out]
        n110 = call-poly <vilib>:"NT Read Value.vi"("Name"="DB/Shoot Toggle") -> ("Boolean"=→"Shoot Toggle":bool)  [unwired: 9 in, 1 out]
        n111 = call-poly <vilib>:"NT Read Value.vi"("Default Value"=FALSE, "Name"="DB/Gear In") -> ("Boolean"=w156:bool)  [unwired: 8 in, 1 out]
        "Gear Status" <- w156
        n112 = call-poly <vilib>:"NT Read Value.vi"("Default Value"=FALSE, "Name"="DB/Pixy Stat") -> ("Boolean"=→"Pixy Object Stat":bool)  [unwired: 8 in, 1 out]
        n113 = local read "NT Connection"() -> (w193:bool)
        n114 = call-poly <vilib>:"NT Write Value.vi"("Numeric"="Slow Turn", "Name"="DB/Slow Turn") -> ()  [unwired: 9 in, 1 out]
        n115 = call-poly <vilib>:"NT Read Value.vi"("Name"="DB/Gear Plate") -> ("Boolean"=→"Gear Plate":bool)  [unwired: 9 in, 1 out]
        n116 = property on="RPM 1" class="DigNum (strict)"("NumText.BGColor"=w274) -> ()  [unwired: 2 in, 2 out]
        n117 = property on="RPM 3" class="DigNum (strict)"("NumText.BGColor"=w272) -> ()  [unwired: 2 in, 2 out]
        n118 = property on="RPM 4" class="DigNum (strict)"("NumText.BGColor"=w271) -> ()  [unwired: 2 in, 2 out]
        n119 = property on="RPM 2" class="DigNum (strict)"("NumText.BGColor"=w273) -> ()  [unwired: 2 in, 2 out]
        n120 = call-poly <vilib>:"NT Write Value.vi"("Numeric"="Pixy Center", "Name"="DB/Pixy Center") -> ()  [unwired: 9 in, 1 out]
        n121 = local read "Auto Array"() -> (w215:string[][])
        n122 = case shown="True" "Update Sheet" {
          tunnel: "Auto Array File Path" -> [_ w459]
          tunnel: w215 -> [_ w458]
          tunnel: [FALSE ("Saved to Sheet") TRUE ("Saved to Sheet")] -> w219
          frame False {
          }
          frame True {
            n123 = call-poly <vilib>:"Write Delimited Spreadsheet.vi"("file path (dialog if empty)"=w459, "2D data"=w458, "delimiter (\\t)"="," ("delimiter (\\t)")) -> ()  [unwired: 11 in, 2 out]
          }
        }
        "Saved to Sheet" <- w219
        n124 = Not(x=w193) -> (.not. x?=w381:bool)
        n125 = And(x="Read Sheet", y="ARM Overwrite") -> (x .and. y?=w222:bool)
        n126 = call-poly <vilib>:"NT Read Value.vi"("Default Value"=FALSE, "Name"="DB/Gear Orient") -> ("Boolean"=w157:bool)  [unwired: 8 in, 1 out]
        n127 = call-poly <vilib>:"NT Read Value.vi"("Name"="DB/Shoot RPM") -> ("Numeric"=→"Shoot RPM":dbl)  [unwired: 9 in, 1 out]
        n128 = call-poly <vilib>:"NT Read Value.vi"("Default Value"=FALSE, "Name"="DB/Gear Lift Stat") -> ("Boolean"=w171:bool)  [unwired: 8 in, 1 out]
        n129 = local read "Auto Array"() -> (w225:string[][])
        n130 = call "Elapsed Time"("Time Target (s)"=0.5, "Reset"=w381, "Auto Reset"=w381) -> ("Time has Elapsed"=w374:bool)  [unwired: 9 in, 7 out]
        n131 = case shown="True" w222 {
          tunnel: "Auto Array File Path" -> [_ w454]
          frame False {
          }
          frame True {
            n132 = call-poly <vilib>:"Read Delimited Spreadsheet.vi"("file path (dialog if empty)"=w454, "delimiter (\\t)"="," ("delimiter (\\t)")) -> ("all rows"=w455:string[][])  [unwired: 8 in, 5 out]
            n133 = local write "ARM Overwrite"(FALSE ("Update\nDB Table")) -> ()
            n134 = local write "Auto Array"(w455) -> ()
          }
        }
        n135 = call-poly <vilib>:"NT Read Value.vi"("Name"="DB/Lift Toggle") -> ("Boolean"=w114:bool)  [unwired: 9 in, 1 out]
        n136 = call-poly <vilib>:"NT Read Value.vi"("Name"="DB/Pixy X") -> ("Numeric"=→"Pixy X":dbl)  [unwired: 9 in, 1 out]
        n137 = case shown="True" w157 {
          tunnel: w156 -> [_ w425]
          tunnel: [FALSE w424] -> w155
          frame False {
          }
          frame True {
            n138 = Not(x=w425) -> (.not. x?=w424:bool)
          }
        }
        n139 = Select(t=6.0, s=w114, f=0.0) -> (s? t:f=w118:dbl)
        n140 = call-poly <vilib>:"NT Write Value.vi"("Numeric"="Auto Turn Speed", "Name"="DB/Auto Turn Speed") -> ()  [unwired: 9 in, 1 out]
        n141 = call-poly <vilib>:"NT Read Value.vi"("Default Value"=FALSE, "Name"="DB/Gear Grab Stat") -> ("Boolean"=w170:bool)  [unwired: 8 in, 1 out]
        n142 = call-poly <vilib>:"NT Read Value.vi"("Name"="DB/Pixy Width") -> ("Numeric"=→"Pixy Width":dbl)  [unwired: 9 in, 1 out]
        n143 = call-poly <vilib>:"NT Read Value.vi"("Name"="DB/Pixy Height") -> ("Numeric"=→"Pixy Height":dbl)  [unwired: 9 in, 1 out]
        n144 = And(x=w374, y=w193) -> (x .and. y?=w373:bool)
        "Auto Ready" <- w373
        n145 = Reshape Array(w225, 250 ("dimension size")) -> (w244:string[])
        n146 = case shown="False" w193 {
          tunnel: [cluster{u32, u32}[] [{16711680, 0}, {35118, 0}] ("Colors [4]") cluster{u32, u32}[] [{16711680, 0}, {15751679, 0}] ("Colors [4]")] -> w194
          frame True {
          }
          frame False {
          }
        }
        n147 = And(x=w170, y=w171) -> (x .and. y?=w173:bool)
        n148 = call-poly <vilib>:"NT Read Value.vi"("Default Value"=FALSE, "Name"="DB/Gear in Lift") -> ("Boolean"=w158:bool)  [unwired: 8 in, 1 out]
        n149 = Select(t=5.0, s=w158, f=w118) -> (s? t:f=w162:dbl)
        n150 = Select(t=1.0, s=w157, f=w162) -> (s? t:f=w182:dbl)
        n151 = Select(t=2.0, s=w171, f=w182) -> (s? t:f=w183:dbl)
        n152 = Select(t=3.0, s=w170, f=w183) -> (s? t:f=w174:dbl)
        n153 = Select(t=4.0, s=w173, f=w174) -> (s? t:f=w175:dbl)
        n154 = call-poly <vilib>:"NT Write Value.vi"("Numeric"="Fast Drive", "Name"="DB/Fast Drive") -> ()  [unwired: 9 in, 1 out]
        n155 = call-poly <vilib>:"NT Write Value.vi"("String Array"=w244, "Name"="DB/Auto Array") -> ()  [unwired: 9 in, 1 out]
        n156 = call-poly <vilib>:"NT Write Value.vi"("Numeric"="Slow Drive", "Name"="DB/Slow Drive") -> ()  [unwired: 9 in, 1 out]
        n157 = case shown="6" w175 {
          tunnel: [cluster{u32, u32}[] [{10420227, 0}, {4345855, 0}] ("Colors [4]") cluster{u32, u32}[] [{10420227, 0}, {6618880, 0}] ("Colors [4]") cluster{u32, u32}[] [{14500607, 0}, {14500607, 0}] ("Colors [4]") cluster{u32, u32}[] [{4385023, 0}, {4385023, 0}] ("Colors [4]") cluster{u32, u32}[] [{12189440, 0}, {12189440, 0}] ("Colors [4]") cluster{u32, u32}[] [{16776305, 0}, {16776305, 0}] ("Colors [4]") cluster{u32, u32}[] [{16739840, 0}, {4345855, 0}] ("Colors [4]")] -> w295
          frame 0, Default {
          }
          frame 1 {
          }
          frame 2 {
          }
          frame 3 {
          }
          frame 4 {
          }
          frame 5 {
          }
          frame 6 {
          }
        }
        n158 = local read "Config Cluster"() -> (w143:T6)
        n159 = property on="Notifyer" class="Bool (strict)"("Colors [4]"=w194) -> ()  [unwired: 2 in, 2 out]
        n160 = property on="Gear Status" class="Bool (strict)"("Blinking"=w155) -> ()  [unwired: 2 in, 2 out]
        n161 = call-poly <vilib>:"NT Read Value.vi"("Name"="DB/PDP") -> ("Numeric Array"=w335:dbl[])  [unwired: 9 in, 1 out]
        n162 = property on="Gear Status" class="Bool (strict)"("Colors [4]"=w295) -> ()  [unwired: 2 in, 2 out]
        n163 = call-poly <vilib>:"NT Read Value.vi"("Default Value"=0.0, "Name"="DB/Tele Time") -> ("Numeric"=w356:dbl)  [unwired: 8 in, 1 out]
        n164 = call-poly <vilib>:"NT Read Value.vi"("Name"="DB/PDP Fault") -> ("Boolean Array"=w242:bool[])  [unwired: 9 in, 1 out]
        n165 = Unbundle By Name(w143) -> ("a"=w138:dbl, "b"=w137:dbl, "c"=w136:dbl, "d"=w135:dbl, "h"=w134:dbl, "proportional gain (Kc)"=w130:dbl, "integral time (Ti, min)"=w128:dbl, "derivative time (Td, min)"=w127:dbl, "Fast Speed"=w126:dbl, "setpoint"=w125:dbl, "Approach Speed"=w124:dbl, "proportional gain (Kc) 2"=w122:dbl, "integral time (Ti, min) 2"=w121:dbl, "derivative time (Td, min) 2"=w120:dbl, "Cutoff Delay"=w111:dbl, "Sense Delay"=w110:dbl, "Wait Till Shoot"=w109:dbl, "proportional gain (Kc) 3"=w104:dbl, "integral time (Ti, min) 3"=w103:dbl, "derivative time (Td, min) 3"=w102:dbl, "Aim Offset"=w106:dbl, "PWM Offset"=w105:dbl)
        n166 = Equal?(x="Auto Select", y="Testing") -> (x = y?=w206:bool)
        n167 = Equal?(x="Position", y="Default") -> (x = y?=w208:bool)
        n168 = Equal?(x="Position", y="Core") -> (x = y?=w207:bool)
        n169 = Equal?(x="Auto Select", y="Default") -> (x = y?=w205:bool)
        n170 = Subtract(x=135.0, y=w356) -> (x-y=w260:dbl)
        "Time Remaining" <- w260
        n171 = Index Array(array=w335) -> (element #1=→"Channel 0":dbl, element #2=→"Channel 1":dbl, element #3=→"Channel 2":dbl, element #4=→"Channel 3":dbl, element #5=→"Channel 4":dbl, element #6=→"Channel 5":dbl, element #7=→"Channel 6":dbl, element #8=→"Channel 7":dbl, element #9=→"Channel 8":dbl, element #10=→"Channel 9":dbl, element #11=→"Channel 10":dbl, element #12=→"Channel 11":dbl, element #13=→"Channel 12":dbl, element #14=→"Channel 13":dbl, element #15=→"Channel 14":dbl, element #16=→"Channel 15":dbl)  [unwired: 16 in]
        n172 = Less?(x=w260, y=45.0) -> (x < y?=w261:bool)
        n173 = Build Array(w208, w207, w205, w206) -> (w204:bool[])
        n174 = case shown="0, Default" "Gear Servo Values" {
          tunnel: [w429 w431] -> w250
          tunnel: [w428 w430] -> w249
          tunnel: "Gear Servo Zero A" -> [w429 _]
          tunnel: "Gear Servo Move A" -> [w428 _]
          tunnel: "Gear Servo Zero B" -> [_ w431]
          tunnel: "Gear Servo Move B" -> [_ w430]
          frame 0, Default {
          }
          frame 1 {
          }
        }
        "Zero" <- w250
        "Move" <- w249
        n175 = Less?(x=w260, y=20.0) -> (x < y?=w262:bool)
        n176 = Less Or Equal To 0?(x=w260) -> (x <= 0?=w266:bool)
        n177 = Or Array Elements(Boolean array=w204) -> (logical OR=w203:bool)
        n178 = Index Array(array=w242) -> (element #1=→"Channel 0":bool, element #2=→"Channel 1":bool, element #3=→"Channel 2":bool, element #4=→"Channel 3":bool, element #5=→"Channel 4":bool, element #6=→"Channel 5":bool, element #7=→"Channel 6":bool, element #8=→"Channel 7":bool, element #9=→"Channel 8":bool, element #10=→"Channel 9":bool, element #11=→"Channel 10":bool, element #12=→"Channel 11":bool, element #13=→"Channel 12":bool, element #14=→"Channel 13":bool, element #15=→"Channel 14":bool, element #16=→"Channel 15":bool)  [unwired: 16 in]
        n179 = Select(t=1.0, s=w261, f=0.0) -> (s? t:f=w264:dbl)
        n180 = call-poly <vilib>:"NT Write Value.vi"("Numeric"="Auto Gear Timeout", "Name"="DB/Gear Timeout") -> ()  [unwired: 9 in, 1 out]
        n181 = Select(t=2.0, s=w262, f=w264) -> (s? t:f=w265:dbl)
        n182 = Equal?(x=w260, y=135.0) -> (x = y?=w358:bool)
        n183 = Less Or Equal To 0?(x=w260) -> (x <= 0?=w359:bool)
        n184 = Select(t=3.0, s=w266, f=w265) -> (s? t:f=w267:dbl)
        n185 = Or(x=w359, y=w358) -> (x .or. y?=w199:bool)
        n186 = And(x=w199, y=w203) -> (x .and. y?=w200:bool)
        n187 = case shown="0, Default" w267 {
          tunnel: [u32 13816530 u32 16769536 u32 16722494 u32 16728814] -> w254
          frame 0, Default {
          }
          frame 1 {
          }
          frame 2 {
          }
          frame 3 {
          }
        }
        n188 = property on="Auto Ready" class="Bool (strict)"("Blinking"=w200) -> ()  [unwired: 2 in, 2 out]
        n189 = Not(x=w193) -> (.not. x?=w284:bool)
        n190 = call-poly <vilib>:"NT Write Value.vi"("Numeric"=w250, "Name"="DB/Gear Zero") -> ()  [unwired: 9 in, 1 out]
        n191 = Or(x=w199, y=w284) -> (x .or. y?=w283:bool)
        n192 = Select(t="Auto Select", s=w373, f=w375) -> (s? t:f=w377:string)
        n193 = Select(t="Position", s=w373, f=w375) -> (s? t:f=w376:string)
        n194 = Build Array(w138, w137, w136, w135, w134) -> (w132:dbl[])
        n195 = Build Array(w130, w128, w127, w126, w125, w124) -> (w129:dbl[])
        n196 = Build Array(w122, w121, w120, w111, w110, w109) -> (w119:dbl[])
        n197 = Build Array(w104, w103, w102) -> (w100:dbl[])
        n198 = property on="Time Remaining" class="DigNum (strict)"("NumText.BGColor"=w254) -> ()  [unwired: 2 in, 2 out]
        n199 = case shown="True" w283 {
          frame False {
            n200 = local write "Time Remain"(FALSE ("Time Remain")) -> ()
          }
          frame True {
            n201 = Not(x="Time Remain") -> (.not. x?=w474:bool)
            n202 = call "Elapsed Time2"("Time Target (s)"=3.0, "Reset"=w474, "Auto Reset"=w474) -> ("Time has Elapsed"=w470:bool)  [unwired: 9 in, 7 out]
            n203 = call "Elapsed Time3"("Time Target (s)"=3.0, "Reset"="Time Remain", "Auto Reset"="Time Remain") -> ("Time has Elapsed"=w469:bool)  [unwired: 9 in, 7 out]
            n204 = Or(x=w470, y=w469) -> (x .or. y?=w471:bool)
            n205 = case shown="True" w471 {
              frame False {
              }
              frame True {
                n206 = local read "Time Remain"() -> (w477:bool)
                n207 = Not(x=w477) -> (.not. x?=w476:bool)
                n208 = local write "Time Remain"(w476) -> ()
              }
            }
          }
        }
        n209 = call-poly <vilib>:"NT Write Value.vi"("String"=w377, "Name"="DB/Auto Select") -> ()  [unwired: 9 in, 1 out]
        n210 = call-poly <vilib>:"NT Write Value.vi"("String"=w376, "Name"="DB/Auto Position") -> ()  [unwired: 9 in, 1 out]
        n211 = call-poly <vilib>:"NT Write Value.vi"("Numeric"=w249, "Name"="DB/Gear Move") -> ()  [unwired: 9 in, 1 out]
        n212 = call-poly <vilib>:"NT Read Value.vi"("Default Value"=w343, "Name"="DB/Notify") -> ("String"=w362:string)  [unwired: 8 in, 1 out]
        n213 = call-poly <vilib>:"NT Write Value.vi"("Numeric"=w105, "Name"="DB/Shoot Offset") -> ()  [unwired: 9 in, 1 out]
        n214 = call-poly <vilib>:"NT Write Value.vi"("Numeric Array"=w132, "Name"="DB/Shoot Equation") -> ()  [unwired: 9 in, 1 out]
        n215 = call-poly <vilib>:"NT Write Value.vi"("Numeric Array"=w129, "Name"="DB/Gear Aimming Config") -> ()  [unwired: 9 in, 1 out]
        n216 = call-poly <vilib>:"NT Write Value.vi"("Numeric Array"=w119, "Name"="DB/Shooting Config") -> ()  [unwired: 9 in, 1 out]
        n217 = Select(t=w362, s=w193, f=w343) -> (s? t:f=w301:string)
        "Notify 2" <- w301
        n218 = call-poly <vilib>:"NT Write Value.vi"("Numeric"=w106, "Name"="DB/Aim Offset") -> ()  [unwired: 9 in, 1 out]
        n219 = call-poly <vilib>:"NT Read Value.vi"("Default Value"=w370, "Name"="DB/Auto Verify") -> ("String"=w371:string)  [unwired: 8 in, 1 out]
        n220 = call-poly <vilib>:"NT Write Value.vi"("Numeric Array"=w100, "Name"="DB/Shoot PID Config") -> ()  [unwired: 9 in, 1 out]
        n221 = Equal?(x=w301, y="NT Connected") -> (x = y?=w340:bool)
        "Notifyer" <- w340
        n222 = Not(x=w340) -> (.not. x?=w342:bool)
        n223 = property on="Notifyer" class="Bool (strict)"("Blinking"=w342) -> ()  [unwired: 2 in, 2 out]
        n224 = Select(t=w371, s=w193, f=w370) -> (s? t:f=→"Verify 2":string)
        n225 = call-poly <vilib>:"NT Write Value.vi"("Numeric"="Lock Servo A", "Name"="DB/Intake Servo A") -> ()  [unwired: 9 in, 1 out]
        n226 = call-poly <vilib>:"NT Write Value.vi"("Numeric"="Lock Servo B", "Name"="DB/Intake Servo B") -> ()  [unwired: 9 in, 1 out]
      }
    }
  }
  n227 = Bundle("Camera Image"=w52, "Dashboard Tab"=w51, "Background"=w47, "Rec Mode"=w38, "Test Slider"=w37, "On/Off"=w36, "Test Ring"=w35, "Rev/Fwd"=w34, "Test Name"=w40, "Motor"=w39, "Progress"=w33, "CheckList"=w43, "Tree"=w42, "Test Tree"=w41, "Command Params"=w27, "Command Selection"=w24, "Execute Command"=w26, "Cmd Status"=w20, "Camera Settings"=w16, "Camera Name"=w15, "Camera Info"=w14, "Camera Settings Right"=w4, "Camera Name Right"=w3, "Camera Image Right"=w2) -> (w44:T19)  [unwired: 1 in]
  n228 = register-events(refnum<vi> refnum, w21) -> (reference out=w61:refnum<event-registration>, error out=w60:errorcluster)  [unwired: 2 in]
  n229 = call "Initialize Camera and CheckList.vi"("ListBox in"=w43) -> ()  [unwired: 11 in]
  n230 = call "Adjust Dashboard Window.vi"("Sizing Refnums"=w44, "Size Constraints"=w48, "VI"=w56, "WIn Mode"=w30) -> ()  [unwired: 8 in]
  n231 = call "Handle Camera Configuration.vi"("CameraNameRef"=w7, "Camera File Name"="Right", "ClusterRef"=w8) -> ()  [unwired: 9 in]
  n232 = vi-ref "Playback Controls.vi"() -> (w62:refnum<vi>)
  n233 = property class="VI"() -> ("Panel"=w64:refnum<vi>)  [unwired: 2 in, 2 out]
  n234 = while {
    tunnel: w72 -> [w487]
    tunnel: w71 -> [_]
    tunnel: [w488] -> _
    i -> [w488]
    stop <- FALSE stop-if-true
    # "Optionally read the DB image,\nlog, or retrieve images from a\nlogged match"
    n235 = local read "Rec Mode"() -> (w483:enum32{"Stop", "Record", "Playback"})
    n236 = local read "Robot IP"() -> (w482:string)
    n237 = call <vilib>:"WPI_CameraRead MJPG for Dashboard.vi"("Camera Settings"="Camera Settings", "Rec Mode"=w483, "Robot IP"=w482, "Camera Name"="Camera Name", "Refnum in"=w487) -> ("Active"=w485:bool, "Refnum out"=w486:T5, "FPS"=w484:dbl, "Bandwidth (Mbps)"=w481:dbl)  [unwired: 3 in]
    n238 = case shown="True" w485 {
      tunnel: w486 -> [w490 w501]
      tunnel: w481 -> [_ w498]
      tunnel: w484 -> [_ w499]
      tunnel: [w490 w495] -> w478
      frame False {
        w492 = u32 1985280 ("Color Box")
        # "Sleep for 500ms"
        n239 = Bundle("Color Box"=w492, "Color Box"=w492) -> (w493:cluster{"Color Box":u32, "Color Box":u32})  [unwired: 1 out]
        n240 = Build Array(w493) -> (w491:cluster{"Color Box":u32, "Color Box":u32}[])
        n241 = property on="Mbps LED" class="Bool (strict)"("Colors [4]"=w491) -> ()  [unwired: 2 in, 2 out]
        n242 = Wait Until Next ms Multiple(millisecond multiple=u32 500) -> ()  [unwired: 1 out]
      }
      frame True {
        # "Here is where you would annotate,\npossibly process, and display the image"
        # "Update Mbps LED"
        n243 = case shown="Default" w498 {
          tunnel: [u32 6618880 ("Color Box") u32 16776722 ("Color Box") u32 16716800 ("Color Box")] -> w502
          frame Default {
          }
          frame 4, 5 {
          }
          frame 6.. {
          }
        }
        n244 = call "IMAQ Clear Overlay"("Image"=w501) -> ("error out"=w504:errorcluster, "Image Out"=w495:T5)  [unwired: 2 in, 7 out]
        n245 = Bundle(FALSE, "Bandwidth (Mbps)"=w498, "FPS"=w499) -> (→"Camera Info":cluster{bool, "Bandwidth (Mbps)":dbl, "FPS":dbl})  [unwired: 1 in]
        n246 = Bundle("Color Box"=w502, "Color Box"=w502) -> (w503:cluster{"Color Box":u32, "Color Box":u32})  [unwired: 1 out]
        n247 = Unbundle By Name(w504) -> ("status"=w505:bool)
        n248 = Build Array(w503) -> (w500:cluster{"Color Box":u32, "Color Box":u32}[])
        n249 = property on="Image Message" class="Str"("Visible"=w505) -> ()  [unwired: 2 in, 2 out]
        n250 = property on="Mbps LED" class="Bool (strict)"("Colors [4]"=w500) -> ()  [unwired: 2 in, 2 out]
      }
    }
    "Camera Image" <- w478
  }
  n251 = while {
    tunnel: w10 -> [w519]
    tunnel: w9 -> [_]
    tunnel: [w513] -> _
    i -> [w513]
    stop <- FALSE stop-if-true
    n252 = local read "Rec Mode"() -> (w517:enum32{"Stop", "Record", "Playback"})
    n253 = local read "Robot IP"() -> (w518:string)
    n254 = call <vilib>:"WPI_CameraRead MJPG for Dashboard.vi"("Camera Settings"="Camera Settings Right", "Rec Mode"=w517, "Robot IP"=w518, "Camera Name"="Camera Name Right", "Refnum in"=w519) -> ("Active"=w512:bool, "Refnum out"=w515:T5, "FPS"=w510:dbl, "Bandwidth (Mbps)"=w511:dbl)  [unwired: 3 in]
    n255 = case shown="False" w512 {
      tunnel: w515 -> [w521 w523]
      tunnel: w511 -> [_ _]
      tunnel: w510 -> [_ _]
      tunnel: [w521 w523] -> w509
      frame False {
        n256 = Wait Until Next ms Multiple(millisecond multiple=u32 500) -> ()  [unwired: 1 out]
      }
      frame True {
      }
    }
    "Camera Image Right" <- w509
  }
  n257 = while {
    tunnel: w53 -> [w535]
    tunnel: w31 -> [w533]
    tunnel: [w531] -> _
    tunnel: u32 1000 ("milliseconds to wait") -> [w530]
    tunnel: w21 -> [w524]
    i -> [w531]
    stop <- FALSE stop-if-true
    n258 = local read "Rec Mode"() -> (w526:enum32{"Stop", "Record", "Playback"})
    n259 = Wait on Notification(notifier=w533, timeout in ms (-1)=w530) -> (notification=w532:string, timed out?=w528:bool)  [unwired: 2 in, 2 out]
    n260 = Equal?(x=w526, y=u16 2 ("Rec Mode")) -> (x = y?=w527:bool)
    n261 = Compound Arithmetic op=OR(invert w528, w527) -> (w529:bool)
    n262 = case shown="True" w529 {
      tunnel: w535 -> [_ w538]
      tunnel: w532 -> [_ w537]
      tunnel: w524 -> [_ w536]
      frame False {
      }
      frame True {
        n263 = call <vilib>:"Bind Controls to SmartDashboard.vi"("RPC ref"=w536, "Bound Control Refs"=w538, "Server IP Address"=w537) -> ()  [unwired: 9 in]
      }
    }
  }
  n264 = property class="Pnl"(reference=w64) -> ("Panes[]"=w65:refnum<vi>[])  [unwired: 1 in, 2 out]
  n265 = Index Array(array=w65) -> (element=w63:refnum<vi>)  [unwired: 1 in]
  n266 = control-ref of="Test Tree"() -> (w66:refnum<vi>)
  n267 = while {
    tunnel: [w548] -> _
    tunnel: w66 -> [w547]
    tunnel: w62 -> [w546]
    tunnel: w61 -> [w545]
    tunnel: w60 -> [_]
    tunnel: w56 -> [w544]
    tunnel: w21 -> [w543]
    tunnel: w19 -> [w542]
    shift-right: [w541] -> _
    shift-left: _ -> [w540]
    tunnel: w13 -> [w539]
    i -> [w548]
    stop <- FALSE stop-if-true
    n268 = event shown="[0] Timeout" {
      selector: w545 -> [_ _ _ _ _ _ _ _ _ _ _ _ _ _ _ _ _ _ _]
      dyn-events: [_ _ _ _ _ _ _ _ _ _ _ _ _ _ w798 _ _ _ _] -> _
      timeout: u32 60 ("milliseconds to wait") -> [_ _ _ _ _ _ _ _ _ _ _ _ _ _ _ _ _ _ _]
      tunnel: w547 -> [w560 _ _ _ _ _ _ _ _ _ _ _ _ _ _ _ _ _ _]
      tunnel: "Test Tree" -> [_ _ _ _ _ _ _ _ _ w765 w773 w775 w779 w787 _ _ _ _ _]
      tunnel: w546 -> [_ _ _ _ _ _ _ _ _ _ _ _ _ _ w800 _ w818 _ _]
      tunnel: w544 -> [_ _ _ _ _ _ _ _ _ _ _ _ _ _ w796 _ _ _ _]
      tunnel: w543 -> [_ _ _ _ _ _ _ _ _ _ _ _ _ _ w792 _ _ _ _]
      tunnel: w542 -> [w555 _ _ _ w716 _ _ _ _ _ _ _ _ _ _ _ _ _ _]
      tunnel: [w554 w599 w701 w706 w714 w723 w733 w740 w752 w764 w771 w774 w778 w786 w791 w813 w815 w819 w830] -> w541
      tunnel: w540 -> [w554 w599 w701 w706 w714 _ _ w740 w752 w764 w771 w774 w778 w786 w791 w813 w815 w819 w830]
      tunnel: w539 -> [w552 _ _ _ _ _ _ _ _ _ _ _ _ _ _ _ _ _ _]
      event Timeout {
        n269 = event-data() -> ()  [unwired: 1 in, 1 out]
        n270 = local read "Mode"() -> (w557:T4)
        n271 = case shown="\"Drive\"" "Dashboard Tab" {
          tunnel: w560 -> [_ _ w576 _ _]
          tunnel: "/TestMode/Automatic/" ("Name Pattern") -> [_ _ w575 _ _]
          tunnel: T20 [{"Operation"=enum."Clear", "Color Box"=14013909}, {"Operation"=enum."Clear", "Color Box"=14013909}, {"Operation"=enum."Clear", "Color Box"=14013909}, {"Operation"=enum."Clear", "Color Box"=14013909}, {"Operation"=enum."Update", "Color Box"=14013909}, {"Operation"=enum."Update", "Color Box"=16777215}, {"Operation"=enum."Clear", "Color Box"=14013909}, {"Operation"=enum."Clear", "Color Box"=14013909}, {"Operation"=enum."Clear", "Color Box"=14013909}] -> [_ _ w568 _ w592]
          tunnel: w557 -> [_ _ w567 _ w591]
          tunnel: u32[] [15790320, 15790320, 15790320, 15790320, 16777215, 16777215, 15790320, 15790320, 15790320] -> [_ _ _ _ w597]
          tunnel: w555 -> [_ _ _ _ w585]
          tunnel: w552 -> [_ w562 _ _ _]
          frame "PDP", Default {
          }
          frame "Drive" {
            n272 = call <vilib>:"WPI_DashboardUpdateNames.vi"("Controls on Tab"=w562) -> ()  [unwired: 11 in]
          }
          frame "Test" {
            w574 = -2 ("Active Item:Row Number")
            n273 = Index Array(array=w568, index=w567) -> (element=w569:T23)
            n274 = Unbundle(w569) -> ("Operation"=w570:enum16{"Update", "Clear"}, "Color Box"=w571:u32)
            n275 = call <vilib>:"NT Read String.vi"("Name"="/TestMode/TestName") -> ("String"=w565:string)  [unwired: 9 in, 1 out]
            n276 = call <vilib>:"NT Read and Format Entries as Tree.vi"("Operation"=w570, "Name Pattern"=w575, "Tree Refnum"=w576) -> ()  [unwired: 7 in, 2 out]
            n277 = case shown="\"\"" w565 {
              tunnel: "/TestMode/TestProgress" ("Name") -> [w578 _]
              tunnel: "/TestMode/TestProgressText" ("Name") -> [w577 _]
              frame Default {
                n278 = call <vilib>:"NT Read Number.vi"("Name"=w578) -> ("Numeric"=w579:dbl)  [unwired: 9 in, 1 out]
                n279 = call <vilib>:"NT Read String.vi"("Name"=w577) -> ("String"=w580:string)  [unwired: 9 in, 1 out]
                n280 = Bundle("Numeric"=w579, "String"=w580) -> (→"Progress":cluster{"Numeric":dbl, "String":string})  [unwired: 1 in]
              }
              frame "" {
                n281 = property on="Progress" class="Clust (strict)"("Visible"=FALSE) -> ()  [unwired: 2 in, 2 out]
                n282 = local write "Test Name"(u16 0) -> ()
              }
            }
            n283 = property on="Test Tree" class="Tree (strict)"("Active Item Row Number"=w574, "ActiveColNum"=w574, "CellBG"=w571, "Active Item Row Number"=-1 ("Active Item:Row Number"), "CellBG"=u32 5789784 ("Color Box")) -> ()  [unwired: 2 in, 2 out]
          }
          frame "Variables" {
            n284 = control-ref of="Tree"() -> (w584:refnum<vi>)
            n285 = call <vilib>:"NT Read and Format Entries as Tree.vi"("Tree Refnum"=w584) -> ()  [unwired: 9 in, 2 out]
          }
          frame "Cmds" {
            w593 = u32 5789784 ("Color Box")
            w594 = T24 {"Row"=-1, "Column"=-2} ("Active Cell:Active Cell")
            w596 = T24 {"Row"=-2, "Column"=-2} ("Active Cell:Active Cell")
            n286 = Index Array(array=w597, index=w591) -> (element=w595:u32)
            n287 = Index Array(array=w592, index=w591) -> (element=w590:T23)
            n288 = Unbundle(w590) -> ("Operation"=w589:enum16{"Update", "Clear"})  [unwired: 1 out]
            n289 = local read "Command Selection"() -> (w588:i32)
            n290 = property on="Command Selection" class="MCListbox (strict)"("ActiveCell"=w596, "CellBG"=w595, "ActiveCell"=w594, "CellBG"=w593) -> ()  [unwired: 2 in, 2 out]
            n291 = call <vilib>:"WPI_DashboardUpdate RPC Info.vi"("Operation"=w589) -> ("update"=w587:bool, "commands"=w586:string[][])  [unwired: 9 in]
            n292 = property on="Command Selection" class="MCListbox (strict)"("ItemNames"=w586) -> ()  [unwired: 2 in, 2 out]
            n293 = property on="Command Params" class="Tbl (strict)"("Active Cell"=w596, "Cell BG Color"=w595, "Active Cell"=w594, "Cell BG Color"=w593) -> ()  [unwired: 2 in, 2 out]
            n294 = call <vilib>:"WPI_DashboardUpdate Command Params.vi"("Update"=w587, "NewVal"=w588, "Commands"=w586, "Param Tbl"=w585) -> ()  [unwired: 7 in, 1 out]
          }
        }
        n295 = call <vilib>:"Connextion Info.vi"() -> ("Connected"=→"NT Connection":bool)  [unwired: 10 in, 1 out]
      }
      event "Test Tree": Value Change {
        # "Show appropriate\ncontrols"
        n296 = event-data() -> ("CtlRef"=w602:refnum<vi>, "NewVal"=w600:string)  [unwired: 1 in]
        n297 = call <vilib>:"WPI_UtilitiesGetTreeIOName.vi"("NewVal"=w600, "TreeControl in"=w602) -> ("I/O Name"=w603:string)  [unwired: 9 in]
        n298 = case shown="\"Camera\"" w603 {
          selector: w603 -> [_ w610 _ w632 w641 _]
          tunnel: w600 -> [_ _ w629 w631 _ w648]
          tunnel: cluster{string[]}[] [{["640x480", "320x240", "160x120"]}, {["Auto", "Fixed indoor", "Fixed outdoor 1", "Fixed outdoor 2", "Fixed fluorescent 1", "Fixed fluorescent 2", "Hold current"]}, {["Auto", "Flicker-free 50 Hz", "Flicker-free 60 Hz", "Hold current"]}, {["None", "Prioritize frame rate", "Prioritize image quality"]}, {["Monochrome", "Color"]}] -> [_ _ _ _ _ w647]
          frame Default {
            w605 = FALSE ("Visible")
            w604 = FALSE ("Visible")
            n299 = property on="Motor" class="Clust (strict)"("Visible"=w604) -> ()  [unwired: 2 in, 2 out]
            n300 = property on="Test Ring" class="Ring (strict)"("Visible"=w604) -> ()  [unwired: 2 in, 2 out]
            n301 = property on="Rev/Fwd" class="Clust (strict)"("Visible"=w605) -> ()  [unwired: 2 in, 2 out]
            n302 = property on="On/Off" class="Bool (strict)"("Visible"=w605) -> ()  [unwired: 2 in, 2 out]
            n303 = property on="Test Slider" class="Slide (strict)"("Visible"=w605) -> ()  [unwired: 2 in, 2 out]
          }
          frame "Analog Out", "Motor", "PWM" {
            w611 = FALSE ("Visible")
            n304 = case shown="\"Analog Out\"" w610 {
              tunnel: [1.0 ("Value") -1.0 ("Value") 0.0 ("Value")] -> w609
              tunnel: [255.0 ("Value") 1.0 ("Value") 5.0 ("Value")] -> w608
              tunnel: [128.0 ("Value") 0.0 ("Value") 0.0 ("Value")] -> w607
              tunnel: [64.0 ("Value") 0.5 ("Value") 1.0 ("Value")] -> w606
              frame "PWM" {
              }
              frame "Motor", Default {
              }
              frame "Analog Out" {
              }
            }
            n305 = property on="Motor" class="Clust (strict)"("Visible"=TRUE) -> ()  [unwired: 2 in, 2 out]
            n306 = property on="Value" class="Slide (strict)"("Value"=w607, "Scale.Minimum"=w609, "Scale.Maximum"=w608, "Scale.Increment"=w606) -> ()  [unwired: 2 in, 2 out]
            n307 = property on="On/Off" class="Bool (strict)"("Visible"=w611) -> ()  [unwired: 2 in, 2 out]
            n308 = property on="Test Slider" class="Slide (strict)"("Visible"=w611) -> ()  [unwired: 2 in, 2 out]
            n309 = property on="Test Ring" class="Ring (strict)"("Visible"=w611) -> ()  [unwired: 2 in, 2 out]
            n310 = property on="Rev/Fwd" class="Clust (strict)"("Visible"=w611) -> ()  [unwired: 2 in, 2 out]
          }
          frame "Servo" {
            w627 = FALSE ("Visible")
            n311 = call <vilib>:"NT Read Number.vi"("Name"=w629) -> ("Numeric"=w628:dbl)  [unwired: 9 in, 1 out]
            n312 = property on="Test Slider" class="Slide (strict)"("Visible"=TRUE, "Scale.Maximum"=170.0 ("Scale.Range:Maximum")) -> ()  [unwired: 2 in, 2 out]
            n313 = local write "Test Slider"(w628) -> ()
            n314 = property on="Motor" class="Clust (strict)"("Visible"=w627) -> ()  [unwired: 2 in, 2 out]
            n315 = property on="Rev/Fwd" class="Clust (strict)"("Visible"=w627) -> ()  [unwired: 2 in, 2 out]
            n316 = property on="On/Off" class="Bool (strict)"("Visible"=w627) -> ()  [unwired: 2 in, 2 out]
            n317 = property on="Test Ring" class="Ring (strict)"("Visible"=w627) -> ()  [unwired: 2 in, 2 out]
          }
          frame "Relay", "Solenoid" {
            w630 = FALSE ("Visible")
            n318 = property on="Motor" class="Clust (strict)"("Visible"=w630) -> ()  [unwired: 2 in, 2 out]
            n319 = property on="Test Slider" class="Slide (strict)"("Visible"=w630) -> ()  [unwired: 2 in, 2 out]
            n320 = Search and Replace String(input string=w631, search string="/Value  **", replace string="/Direction") -> (result string=w637:string)  [unwired: 5 in, 3 out]
            n321 = property on="Test Ring" class="Ring (strict)"("Visible"=w630) -> ()  [unwired: 2 in, 2 out]
            n322 = call <vilib>:"NT Read String.vi"("Name"=w637) -> ("String"=w635:string)  [unwired: 9 in, 1 out]
            n323 = Equal?(x="Both directions", y=w635) -> (x = y?=w633:bool)
            n324 = Not(x=w633) -> (.not. x?=w634:bool)
            n325 = property on="Rev/Fwd" class="Clust (strict)"("Visible"=w633) -> ()  [unwired: 2 in, 2 out]
            n326 = property on="On/Off" class="Bool (strict)"("Visible"=w634, "Caption.Text"=w632) -> ()  [unwired: 2 in, 2 out]
          }
          frame "Compressor", "Digital Out" {
            w640 = FALSE ("Visible")
            # "Get direction and finish"
            n327 = property on="Motor" class="Clust (strict)"("Visible"=w640) -> ()  [unwired: 2 in, 2 out]
            n328 = property on="Test Slider" class="Slide (strict)"("Visible"=w640) -> ()  [unwired: 2 in, 2 out]
            n329 = property on="Test Ring" class="Ring (strict)"("Visible"=w640) -> ()  [unwired: 2 in, 2 out]
            n330 = property on="On/Off" class="Bool (strict)"("Visible"=TRUE, "Caption.Text"=w641) -> ()  [unwired: 2 in, 2 out]
            n331 = property on="Rev/Fwd" class="Clust (strict)"("Visible"=FALSE) -> ()  [unwired: 2 in, 2 out]
          }
          frame "Camera" {
            n332 = call <vilib>:"Get Last Path Segment.vi"("String in"=w648) -> ("String out"=w649:string)  [unwired: 10 in]
            n333 = property on="On/Off" class="Bool (strict)"("Visible"=FALSE) -> ()  [unwired: 2 in, 2 out]
            n334 = property on="Motor" class="Clust (strict)"("Visible"=FALSE) -> ()  [unwired: 2 in, 2 out]
            n335 = property on="Rev/Fwd" class="Clust (strict)"("Visible"=FALSE) -> ()  [unwired: 2 in, 2 out]
            n336 = case shown="\"White Balance  **\"" w649 {
              tunnel: w648 -> [w655 w664 w673 w682 w691 _ w697]
              tunnel: w647 -> [w653 w661 w670 w679 w688 _ _]
              frame "Size  **" {
                n337 = Index Array(array=w653) -> (element=w652:cluster{string[]})  [unwired: 1 in]
                n338 = call <vilib>:"NT Read String.vi"("Name"=w655) -> ("String"=w654:string)  [unwired: 9 in, 1 out]
                n339 = Unbundle(w652) -> (w650:string[])
                n340 = Match First String(2:w650, 3:w654) -> (0:w651:i32)  [unwired: 1 out]
                n341 = property on="Test Ring" class="Ring (strict)"("Value"=w651, "Strings []"=w650) -> ()  [unwired: 2 in, 2 out]
                n342 = property on="Test Ring" class="Ring (strict)"("Visible"=TRUE) -> ()  [unwired: 2 in, 2 out]
                n343 = property on="Test Slider" class="Slide (strict)"("Visible"=FALSE) -> ()  [unwired: 2 in, 2 out]
              }
              frame "White Balance  **" {
                n344 = Index Array(array=w661, index=1) -> (element=w662:cluster{string[]})
                n345 = call <vilib>:"NT Read String.vi"("Name"=w664) -> ("String"=w663:string)  [unwired: 9 in, 1 out]
                n346 = Unbundle(w662) -> (w659:string[])
                n347 = Match First String(2:w659, 3:w663) -> (0:w658:i32)  [unwired: 1 out]
                n348 = property on="Test Ring" class="Ring (strict)"("Value"=w658, "Strings []"=w659) -> ()  [unwired: 2 in, 2 out]
                n349 = property on="Test Ring" class="Ring (strict)"("Visible"=TRUE) -> ()  [unwired: 2 in, 2 out]
                n350 = property on="Test Slider" class="Slide (strict)"("Visible"=FALSE) -> ()  [unwired: 2 in, 2 out]
              }
              frame "Exposure  **" {
                n351 = Index Array(array=w670, index=2) -> (element=w671:cluster{string[]})
                n352 = call <vilib>:"NT Read String.vi"("Name"=w673) -> ("String"=w672:string)  [unwired: 9 in, 1 out]
                n353 = Unbundle(w671) -> (w667:string[])
                n354 = Match First String(2:w667, 3:w672) -> (0:w668:i32)  [unwired: 1 out]
                n355 = property on="Test Ring" class="Ring (strict)"("Value"=w668, "Strings []"=w667) -> ()  [unwired: 2 in, 2 out]
                n356 = property on="Test Ring" class="Ring (strict)"("Visible"=TRUE) -> ()  [unwired: 2 in, 2 out]
                n357 = property on="Test Slider" class="Slide (strict)"("Visible"=FALSE) -> ()  [unwired: 2 in, 2 out]
              }
              frame "Exposure Priority  **" {
                n358 = Index Array(array=w679, index=3) -> (element=w680:cluster{string[]})
                n359 = call <vilib>:"NT Read String.vi"("Name"=w682) -> ("String"=w681:string)  [unwired: 9 in, 1 out]
                n360 = Unbundle(w680) -> (w676:string[])
                n361 = Match First String(2:w676, 3:w681) -> (0:w677:i32)  [unwired: 1 out]
                n362 = property on="Test Ring" class="Ring (strict)"("Value"=w677, "Strings []"=w676) -> ()  [unwired: 2 in, 2 out]
                n363 = property on="Test Ring" class="Ring (strict)"("Visible"=TRUE) -> ()  [unwired: 2 in, 2 out]
                n364 = property on="Test Slider" class="Slide (strict)"("Visible"=FALSE) -> ()  [unwired: 2 in, 2 out]
              }
              frame "Color Enable  **" {
                n365 = Index Array(array=w688, index=4) -> (element=w689:cluster{string[]})
                n366 = call <vilib>:"NT Read String.vi"("Name"=w691) -> ("String"=w690:string)  [unwired: 9 in, 1 out]
                n367 = Unbundle(w689) -> (w685:string[])
                n368 = Match First String(2:w685, 3:w690) -> (0:w686:i32)  [unwired: 1 out]
                n369 = property on="Test Ring" class="Ring (strict)"("Value"=w686, "Strings []"=w685) -> ()  [unwired: 2 in, 2 out]
                n370 = property on="Test Ring" class="Ring (strict)"("Visible"=TRUE) -> ()  [unwired: 2 in, 2 out]
                n371 = property on="Test Slider" class="Slide (strict)"("Visible"=FALSE) -> ()  [unwired: 2 in, 2 out]
              }
              frame Default {
                n372 = property on="Test Ring" class="Ring (strict)"("Visible"=FALSE) -> ()  [unwired: 2 in, 2 out]
                n373 = property on="Test Slider" class="Slide (strict)"("Visible"=FALSE) -> ()  [unwired: 2 in, 2 out]
              }
              frame "Brightness  **", "Color Level  **", "Compression  **", "FPS  **", "Sharpness  **" {
                n374 = call <vilib>:"NT Read Number.vi"("Name"=w697) -> ("Numeric"=w696:dbl)  [unwired: 9 in, 1 out]
                n375 = local write "Test Slider"(w696) -> ()
                n376 = property on="Test Slider" class="Slide (strict)"("Visible"=TRUE, "Scale.Maximum"=100.0 ("Scale.Range:Maximum")) -> ()  [unwired: 2 in, 2 out]
                n377 = property on="Test Ring" class="Ring (strict)"("Visible"=FALSE) -> ()  [unwired: 2 in, 2 out]
              }
            }
          }
        }
        n378 = property on="Progress" class="Clust (strict)"("Visible"=FALSE) -> ()  [unwired: 2 in, 2 out]
      }
      event "Test Name": Mouse Enter {
        # "Populate the ring with the list of tests"
        n379 = event-data() -> ()  [unwired: 1 in, 1 out]
        n380 = call <vilib>:"NT Read String Array.vi"("Name"="/TestMode/TestList") -> ("String Array"=w705:string[])  [unwired: 9 in, 1 out]
        n381 = Build Array (concatenate)("Select the test to run...", w705) -> (w704:string[])
        n382 = property on="Test Name" class="Ring (strict)"("Strings []"=w704) -> ()  [unwired: 2 in, 2 out]
      }
      event "Test Name": Value Change {
        w707 = FALSE ("Visible")
        # "Tell the robot the test name to run"
        n383 = event-data() -> ("NewVal"=w711:u16)  [unwired: 1 in]
        n384 = property on="Test Name" class="Ring (strict)"() -> ("Strings []"=w712:string[])  [unwired: 2 in, 2 out]
        n385 = local write "Progress"(T7 {"Test Progress"=0, "Test Progress Text"=""} ("Progress")) -> ()
        n386 = Index Array(array=w712, index=w711) -> (element=w710:string)
        n387 = call <vilib>:"NT Write String.vi"("String"=w710, "Name"="/TestMode/TestName") -> ()  [unwired: 9 in, 1 out]
        n388 = property on="Progress" class="Clust (strict)"("Visible"=TRUE) -> ()  [unwired: 2 in, 2 out]
        n389 = property on="Motor" class="Clust (strict)"("Visible"=w707) -> ()  [unwired: 2 in, 2 out]
        n390 = property on="Test Slider" class="Slide (strict)"("Visible"=w707) -> ()  [unwired: 2 in, 2 out]
        n391 = property on="On/Off" class="Bool (strict)"("Visible"=w707) -> ()  [unwired: 2 in, 2 out]
        n392 = property on="Rev/Fwd" class="Clust (strict)"("Visible"=w707) -> ()  [unwired: 2 in, 2 out]
        n393 = property on="Test Ring" class="Ring (strict)"("Visible"=w707) -> ()  [unwired: 2 in, 2 out]
      }
      event "Command Selection": Value Change {
        # "Get the params and show in table"
        n394 = event-data() -> ("NewVal"=w717:i32)  [unwired: 1 in]
        n395 = property on="Command Selection" class="MCListbox (strict)"() -> ("ItemNames"=w715:string[][])  [unwired: 2 in, 2 out]
        n396 = call <vilib>:"WPI_DashboardUpdate Command Params.vi"("NewVal"=w717, "Commands"=w715, "Param Tbl"=w716) -> ()  [unwired: 8 in, 1 out]
      }
      event "Execute Command": Value Change {
        # "Started one, Unique ID holds\nresponse"
        n397 = event-data() -> ()  [unwired: 1 in, 1 out]
        n398 = property on="Command Selection" class="MCListbox (strict)"() -> ("ItemNames"=w728:string[][])  [unwired: 2 in, 2 out]
        n399 = Index Array(array=w728, index (row)="Command Selection", index (col)=0) -> (element=w726:string)
        n400 = call <vilib>:"Invoke Commands.vi"("Command Params"="Command Params", "Function Name"=w726) -> ("Params"=w722:u8, "Started"=w721:bool)  [unwired: 7 in, 1 out]
        n401 = Array Subset(array="Command Params", length (row)=w722) -> (w723:string[][])  [unwired: 3 in]
        n402 = Select(t="Executing" ("Cmd Status"), s=w721, f="" ("Cmd Status")) -> (s? t:f=→"Cmd Status":string)
      }
      event "Command Selection": Double Click {
        n403 = event-data() -> ("Row"=w736:i32)  [unwired: 1 in]
        n404 = property on="Command Selection" class="MCListbox (strict)"() -> ("ItemNames"=w739:string[][])  [unwired: 2 in, 2 out]
        n405 = local read "Command Params"() -> (w735:string[][])
        n406 = Index Array(array=w739, index (row)=w736, index (col)=0) -> (element=w737:string)
        n407 = call <vilib>:"Invoke Commands.vi"("Command Params"=w735, "Function Name"=w737) -> ("Params"=w734:u8, "Started"=w729:bool)  [unwired: 7 in, 1 out]
        n408 = Array Subset(array=w735, length (row)=w734) -> (w733:string[][])  [unwired: 3 in]
        n409 = Select(t="Executing" ("Cmd Status"), s=w729, f="" ("Cmd Status")) -> (s? t:f=w730:string)
        n410 = local write "Cmd Status"(w730) -> ()
      }
      event "CheckList": Double Click {
        # "Shift clears all"
        # "Update symbols on the listbox"
        n411 = event-data() -> ("PlatMods.Shift"=w741:bool, "Row"=w743:i32)  [unwired: 1 in]
        n412 = case shown="True" w741 {
          tunnel: w743 -> [w747 _]
          tunnel: 1 -> [w746 _]
          frame False {
            n413 = property on="CheckList" class="LstBox (strict)"() -> ("Item Symbols"=w745:i32[])  [unwired: 2 in, 2 out]
            n414 = Replace Array Subset(array=w745, new element=w746, index=w747) -> (w744:i32[])
            n415 = property on="CheckList" class="LstBox (strict)"("Item Symbols"=w744) -> ()  [unwired: 2 in, 2 out]
          }
          frame True {
            w748 = 0 ("Top Row")
            n416 = property on="CheckList" class="LstBox (strict)"() -> ("Number of Rows"=w750:u32)  [unwired: 2 in, 2 out]
            n417 = Initialize Array(0, w750) -> (w749:i32[])
            n418 = property on="CheckList" class="LstBox (strict)"("Top Row"=w748, "Value"=w748, "Item Symbols"=w749) -> ()  [unwired: 2 in, 2 out]
          }
        }
      }
      event "CheckList": Key Down {
        # "Update symbols on the listbox\nLeft and right keys check and uncheck"
        n419 = event-data() -> ("VKey"=w754:T21)  [unwired: 1 in]
        n420 = case shown="\"Left\", \"Right\"" w754 {
          selector: w754 -> [w759 _]
          tunnel: eventvkey."Left" ("VKey") -> [w757 _]
          frame "Left", "Right" {
            n421 = Equal?(x=w757, y=w759) -> (x = y?=w758:bool)
            n422 = Select(t=0, s=w758, f=1) -> (s? t:f=w760:i32)
            n423 = property on="CheckList" class="LstBox (strict)"() -> ("Item Symbols"=w763:i32[])  [unwired: 2 in, 2 out]
            n424 = Replace Array Subset(array=w763, new element=w760, index="CheckList") -> (w762:i32[])
            n425 = property on="CheckList" class="LstBox (strict)"("Item Symbols"=w762) -> ()  [unwired: 2 in, 2 out]
          }
          frame Default {
          }
        }
      }
      event "Motor.Enable": Value Change {
        # "When the test mode otor enable helper is set, update that\ntree row item's value"
        n426 = event-data() -> ("NewVal"=w769:bool)  [unwired: 1 in]
        n427 = Unbundle("Motor") -> ("Value"=w768:dbl)  [unwired: 1 out]
        n428 = Select(t=w768, s=w769, f=0.0) -> (s? t:f=w766:dbl)
        n429 = call <vilib>:"NT Write Number.vi"("Numeric"=w766, "Name"=w765) -> ()  [unwired: 9 in, 1 out]
      }
      event "Test Slider": Value Change {
        # "When the test mode slider helper is set, update that\ntree row item's value"
        n430 = event-data() -> ("NewVal"=w772:dbl)  [unwired: 1 in]
        n431 = call <vilib>:"NT Write Number.vi"("Numeric"=w772, "Name"=w773) -> ()  [unwired: 9 in, 1 out]
      }
      event "On/Off": Value Change {
        # "When the test mode on/off helper value is set, update that\ntree row item's value"
        n432 = event-data() -> ("NewVal"=w777:bool)  [unwired: 1 in]
        n433 = Boolean To (0,1)(Boolean=w777) -> (0, 1=w776:i16)
        n434 = call <vilib>:"NT Write Number.vi"("Numeric"=w776, "Name"=w775) -> ()  [unwired: 9 in, 1 out]
      }
      event "Rev/Fwd": Value Change {
        # "When the test mode helper value for relays is set, update that\ntree row item's value"
        n435 = event-data() -> ("NewVal.Forward"=w785:bool, "NewVal.Reverse"=w784:bool)  [unwired: 1 in]
        n436 = Boolean To (0,1)(Boolean=w785) -> (0, 1=w781:i16)
        n437 = Boolean To (0,1)(Boolean=w784) -> (0, 1=w783:i16)
        n438 = Negate(x=w783) -> (-x=w782:i16)
        n439 = Add(x=w781, y=w782) -> (x+y=w780:i16)
        n440 = call <vilib>:"NT Write Number.vi"("Numeric"=w780, "Name"=w779) -> ()  [unwired: 9 in, 1 out]
      }
      event "Test Ring": Value Change {
        # "When a test mode helper value is selected from the ring,\nset the tree item's variable to the string value"
        n441 = event-data() -> ("NewVal"=w789:u16)  [unwired: 1 in]
        n442 = property on="Test Ring" class="Ring (strict)"() -> ("Strings []"=w790:string[])  [unwired: 2 in, 2 out]
        n443 = Index Array(array=w790, index=w789) -> (element=w788:string)
        n444 = call <vilib>:"NT Write String.vi"("String"=w788, "Name"=w787) -> ()  [unwired: 9 in, 1 out]
      }
      event "Rec Mode": Value Change {
        # "Update globals for recording mode and path to read log from.\nClear when logging and let NetworkTables set path for vision to\nuse."
        n445 = event-data() -> ("NewVal"=w801:enum32{"Stop", "Record", "Playback"})  [unwired: 1 in]
        n446 = global write "WPI_DashboardLogging Global.vi" "Logging Filename"(path "") -> ()
        n447 = global write "WPI_DashboardLogging Global.vi" "Recording"(w801) -> ()
        n448 = case shown="\"Playback\"" w801 {
          tunnel: w800 -> [_ w803 w812]
          tunnel: [_ _ w811] -> w798
          tunnel: [_ _ w810] -> _
          tunnel: w796 -> [_ _ w808]
          tunnel: cluster{i32, i32} {-250, 170} -> [_ _ w807]
          tunnel: [_ _ T22 {"Image Size"=TRUE, "Image Type"=TRUE, "Pixel Value"=TRUE, "ROI Information"=TRUE, "Zoom Factor"=FALSE} ("Image Information Shown:All Elements")] -> w794
          tunnel: [_ _ TRUE ("Zoom Factor")] -> w793
          tunnel: w792 -> [_ _ w804]
          frame Default {
          }
          frame "Stop", "Record" {
            # "Place Window too"
            n449 = invoke class="VI" method="FP.Close"(reference=w803) -> (reference out=w802:refnum<vi>)  [unwired: 2 in, 2 out]
            n450 = invoke class="VI" method="Abort VI"(reference=w802) -> ()  [unwired: 2 in, 3 out]
          }
          frame "Playback" {
            n451 = call "Open Playback Panel.vi"("Offset"=w807, "DB VI Ref"=w808, "Playback in"=w812) -> ("Playback out"=w809:refnum<vi>)  [unwired: 8 in]
            n452 = register-events(w809, w804) -> (reference out=w811:refnum<event-registration>, error out=w810:errorcluster)  [unwired: 2 in]
          }
        }
        n453 = property on="Camera Image" class="ImageControl"("Image Information Shown"=w794, "Image Information Visible"=w793) -> ()  [unwired: 2 in, 2 out]
        n454 = call <vilib>:"WPI_DashboardNT Log FieldName Cache.vi"("Operation"=enum16{"Lookup/Add", "Index", "Clear"}."Clear") -> ()  [unwired: 8 in, 3 out]
      }
      event Panel Close {
        w814 = enum32{"Stop", "Record", "Playback"}."Stop" ("Rec Mode")
        # "Playback window has been closed, abort"
        n455 = event-data() -> ()  [unwired: 1 in, 4 out]
        n456 = local write "Rec Mode"(w814) -> ()
        n457 = global write "WPI_DashboardLogging Global.vi" "Recording"(w814) -> ()
      }
      event Panel Close {
        # "Abort playback window and ourself"
        n458 = event-data() -> ()  [unwired: 1 in, 4 out]
        n459 = invoke class="VI" method="FP.Close"(reference=w818) -> (reference out=w817:refnum<vi>)  [unwired: 2 in, 2 out]
        n460 = invoke class="VI" method="Abort VI"(reference=w817) -> (error out=w816:errorcluster)  [unwired: 2 in, 2 out]
        n461 = invoke class="VI" method="Abort VI"(error in=w816) -> ()  [unwired: 2 in, 3 out]
      }
      event User Event {
        n462 = event-data() -> ("IDs"=w825:cluster{"RPC field ID":u16, "Unique ID":u16}, "String"=w824:string)  [unwired: 1 in]
        n463 = Bundle("IDs"=w825, "String"=w824) -> (w823:T9)  [unwired: 1 in]
        n464 = call <vilib>:"Retrieve RPC Response.vi"("RPC Response"=w823) -> ("Output"=w821:string[][])  [unwired: 10 in]
        n465 = Build Array (concatenate)(w819, w821) -> (w820:string[][])
        n466 = local write "Command Params"(w820) -> ()
        n467 = local write "Cmd Status"("" ("Cmd Status")) -> ()
      }
      event "Tree": Double Click {
        n468 = event-data() -> ("PlatMods"=w829:T25, "Tag"=w828:string)  [unwired: 1 in]
        n469 = Unbundle(w829) -> ("Shift"=w827:bool)  [unwired: 4 out]
        n470 = Not(x=w827) -> (.not. x?=w826:bool)
        n471 = call <vilib>:"NT Update Persistence.vi"("Persistence"=w826, "Name"=w828) -> ()  [unwired: 9 in, 1 out]
      }
    }
  }
  n472 = while {
    tunnel: w63 -> [w832]
    i -> [w835]
    stop <- FALSE stop-if-true
    n473 = Wait (ms)(milliseconds to wait=u32 100) -> ()  [unwired: 1 out]
    n474 = case shown="\"Playback\"" "Rec Mode" {
      tunnel: w835 -> [_ _ w850]
      tunnel: [u32 2829099 ("Base Color") u32 11141120 ("Target Color") w839] -> w831
      frame "Stop", Default {
        # "Reset the color, extra updates don't cost much"
      }
      frame "Record" {
      }
      frame "Playback" {
        # "Playback"
        n475 = Quotient & Remainder(x=w850, y=u32 50 ("milliseconds to wait")) -> (x-y*floor(x/y)=w846:u32)  [unwired: 1 out]
        n476 = Divide(x=w846, y=u32 50 ("milliseconds to wait")) -> (x/y=w843:dbl)
        n477 = Multiply(x=6.283185307179586, y=w843) -> (x*y=w848:dbl)
        n478 = Sine(x=w848) -> (sin(x)=w847:dbl)
        n479 = Absolute Value(x=w847) -> (abs(x)=w840:dbl)
        n480 = call "Interpolate RGB Color.vi"("Proportion"=w840, "Target Color"=u32 30976, "Base Color"=u32 2829099) -> ("Result Color"=w839:u32)  [unwired: 8 in]
      }
    }
    n481 = property class="Pane"(reference=w832, "PaneColor"=w831) -> ()  [unwired: 1 in, 2 out]
  }
  n482 = local write "Dashboard Tab"(T2."Drive" ("Dashboard Tab")) -> ()
  n483 = property on="On/Off" class="Bool (strict)"("Visible"=w32) -> ()  [unwired: 2 in, 2 out]
  n484 = property on="Motor" class="Clust (strict)"("Visible"=w32) -> ()  [unwired: 2 in, 2 out]
  n485 = property on="Progress" class="Clust (strict)"("Visible"=w32) -> ()  [unwired: 2 in, 2 out]
  n486 = property on="Test Ring" class="Ring (strict)"("Visible"=w32) -> ()  [unwired: 2 in, 2 out]
  n487 = property on="Rev/Fwd" class="Clust (strict)"("Visible"=w32) -> ()  [unwired: 2 in, 2 out]
  n488 = while {
    tunnel: u16 1741 ("timeout ms (25000)") -> [w852]
    stop <- FALSE stop-if-true
    n489 = TCP Create Listener(10:w852) -> (0:w851:errorcluster, 3:w853:refnum<k5>)  [unwired: 4 in, 1 out]
    n490 = case shown="No Error" w851 {
      selector: w851 -> [w855 _]
      tunnel: w853 -> [w856 _]
      frame No Error {
        n491 = while {
          tunnel: w856 -> [w859]
          tunnel: w855 -> [w858]
          stop <- FALSE stop-if-true
          n492 = TCP Wait On Listener(8:w858, 11:w859) -> (0:w860:errorcluster, 4:w861:refnum<k5>)  [unwired: 2 in, 3 out]
          n493 = local write "TCP"(w861) -> ()
          n494 = case shown="No Error" w860 {
            frame No Error {
            }
            frame Error {
              n495 = Wait (ms)(milliseconds to wait=u32 1000) -> ()  [unwired: 1 out]
            }
          }
        }
      }
      frame Error {
        n496 = Wait (ms)(milliseconds to wait=u32 1000) -> ()  [unwired: 1 out]
      }
    }
  }
  n497 = local write "Command Selection"(u16 0 ("milliseconds to wait")) -> ()
  n498 = local write "Command Params"(string[][] [] ("Command Params")) -> ()
  n499 = global write "WPI_DashboardLogging Global.vi" "Recording"(w57) -> ()
  n500 = local write "Rec Mode"(w57) -> ()
